vi "Full_Display.vi"() -> ()   [LabVIEW 2018]
uses:
  <vilib>/Utility/file.llb/Read Delimited Spreadsheet (DBL).vi
  D:/LocalElwood/localElwood/Manuals/SLM/SDK_from_1.1.0.84M/Blink_C_wrapper.dll
panel:
  out "Was it modified?":bool
  in  "stop 3":bool
  in  "stop 2":bool
  out "ok for com 2":bool
  out "new picture":picture
  in  "stop":bool
  in  "exit":bool
  in  "disconnect":bool
  in  "Divergence Button":bool
  in  "Orientation :":enum16{"Auto Orient", "0 Degrees", "45 Degress"}(ring)
  in  "1ovre on":bool
  in  "FWHM On":bool
  in  "Log on":bool
  in  "Gauss on":bool
  in  "1ovre":bool
  in  "FWHM":bool
  in  "Log":bool
  in  "Gauss":bool caption="Press to Activate Measurements"
  in  "Center :":enum16{"Centroid", "Peak"}(ring)
  in  "Display":T1(ring)=enum."3D Display" caption="Press Buttons to Activate XY Measurements"
  in  "Definition :":T2(ring)
  in  "Manual":bool
  in  "subtract background":bool caption="Capture"
  in  "Gray Scale":bool
  in  "mm":dbl=200.0 min=0.0 max=9999999.0
  in  "ms":dbl=50.0 min=0.06 max=200.0 step=0.01
  in  "Auto":bool=TRUE
  in  "Format Image":string(combo)="TXT"
  in  "save current image":bool caption="Capture"
  in  "start capture":bool caption="Capture"
  in  "connect":bool
  out "ok for com":bool
  out "Connected":bool
  out "Camera Serial Number":string
  out "PC Beamage Version":string caption="PC Beamage SW Version"
  out "Y Divergence":string
  out "X Divergence":string
  in  "Y Axis Measurements":T3(ring)=enum."Centroid"
  out "Y Axis Measurement":string caption="Y Axis Centroid"
  out "X Axis Measurement":string caption="X Axis Centroid"
  in  "X Axis Measurements":T3(ring)=enum."Centroid"
  in  "Common Measurements":T4(ring)=enum."Measure Effective Diameter"
  out "Common Measurement":string caption="Effective Diameter"
  in  "Time out":i32=-1
  out "DLL Present":bool=TRUE
  in  "Grating constant D\n    (0.2 by default)":dbl=0.2
  in  "Load angle_intensity":bool
  in  "Save angle_intensity":bool
  in  "main stop":bool
  in  "amp_angles":dbl=0.2
  in  "Order of pitch fork":dbl=1.0
  out "Pattern":picture
  out "File_title":string
  in  "Root Path":path=path "C:/localElwood/LabView/Magnet C006/Display_SLM_with_Zernike_Trigger_Beamprofiler_Bin"
  in  "LUT file location":string="C:\\Program Files\\Meadowlark Optics\\Blink 1920 HDMI\\LUT Files\\linear.blt"
  out "Status":dbl
  out "angle_intensity":dbl[](array[numeric])
  # "1\n2\n3\n4\n5\n6\n7\n8\n9\n10\n11\n12\n13\n14\n15\n16\n17\n18\n19\n20\n21\n22\n23\n24\n25\n26\n27\n28\n29\n30\n31\n32\n33\n34\n35\n36"
  # "* Remember to initialize angle_intensity, 0-1\n* Check the laser power is okay with 200ms fixed exposure time.\n* Check the root path is correct for this computer.\n* Check Z_num is initialized correctly."
  # "0"
  # "1"
  # "2"
  # "3"
  # "4"
  # "5"
  # "6"
  # "7"
  # "8"
  # "9"
  # "10"
  # "11"
  # "12"
  # "13"
  # "14"
  # "amp_angles defines the maximum\nintensity modulation you want to \napply. By default, it's 0.2."
  # "15"
  # "16"
  # "17"
  # "18"
  # "19"
  # "20"
  # "21"
  # "22"
  # "23"
  # "24"
  # "25"
  # "26"
  # "27"
  # "28"
  # "29"
  # "30"
  # "31"
  # "32"
  # "33"
  # "34"
  # "35"
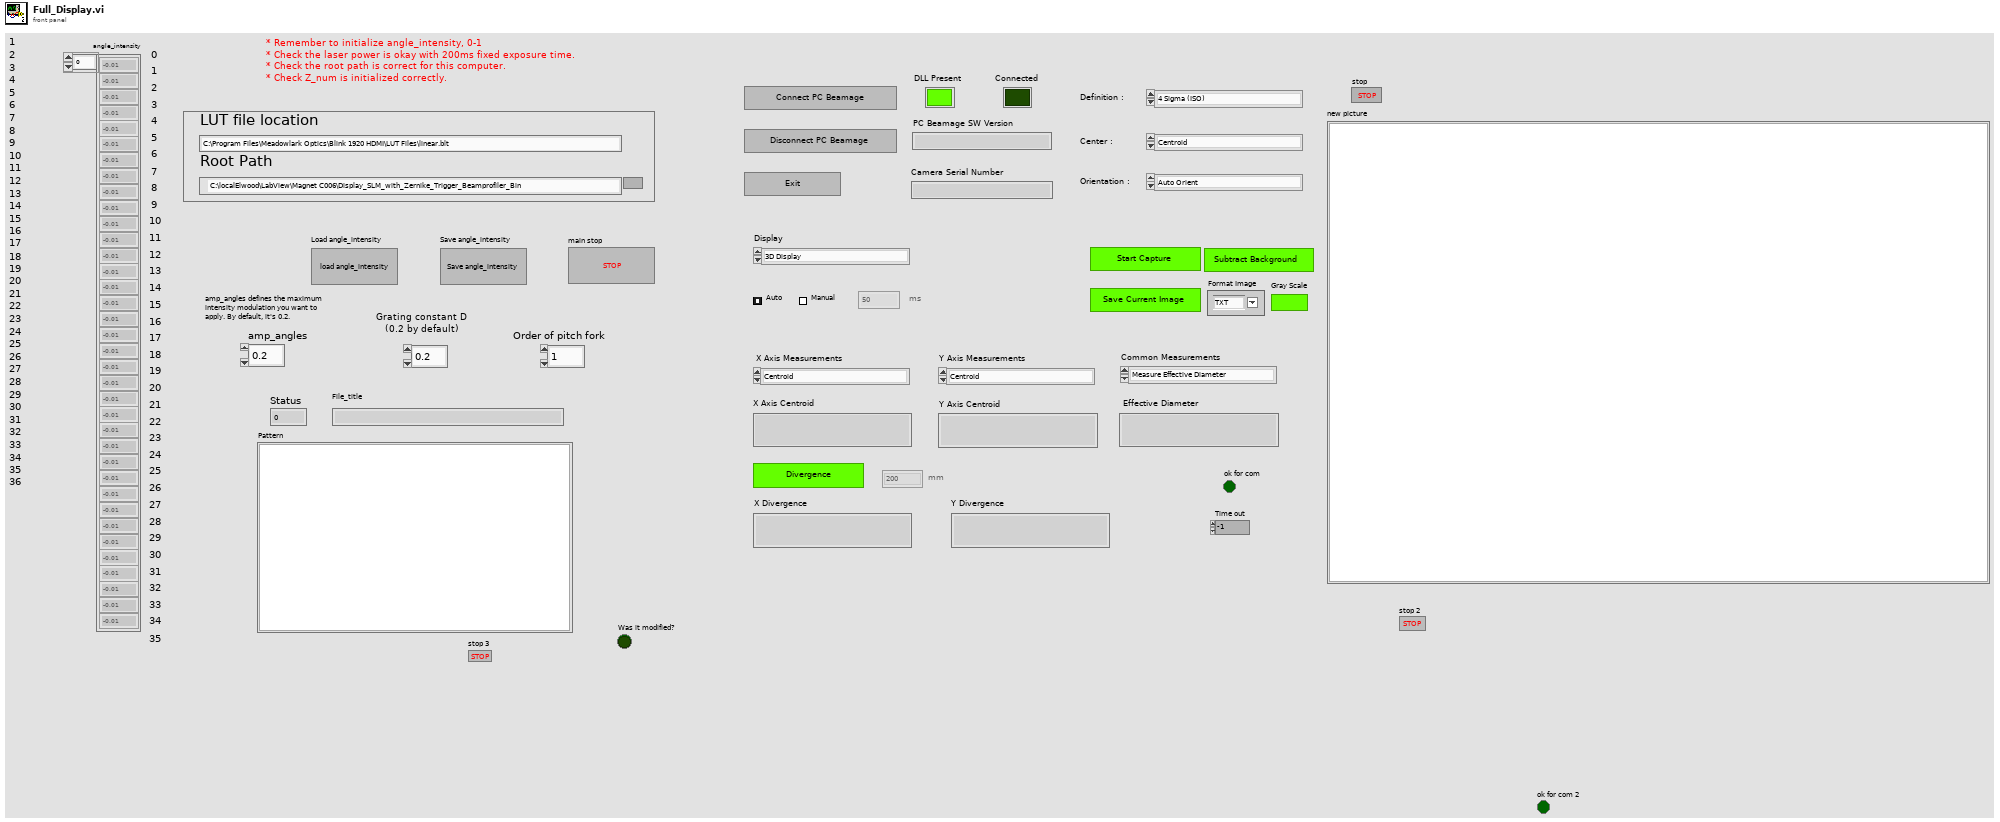
[diagram p1: front panel]
types:
  T1 = enum16{"2D Display", "3D Display", "XY Display", "Beam Track Display"}
  T2 = enum16{"4 Sigma (ISO)", "FWHM along Crosshairs (50%)", "1 / e^2 along Crosshairs (13.5%)", "86 % effective Diameter"}
  T3 = enum16{"1/e^2", "Centroid", "Delta", "FWHM", "Gaussian Equation", "Gaussian % Fit", "Roughness Fit", "Last", "Mean", "Peak to Average Ratio", "Peak"}
  T4 = enum16{"Measure Azimuth", "Measure Delta", "Measure Effective Diameter", "Measure Ellipticity", "Measure Number of Samples", "Measure Orientation", "Measure Peak Saturation", "Measure Minor Axis", "Measure Major Axis", "Measure RMS", ""}
  T5 = enum16{"open", "replace", "create", "open or create", "replace or create", "replace or create with confirmation"}
  T6 = typedef "LVBoundsTypeDef.ctl" = cluster{"Width":u32, "Height":u32}
  T7 = typedef "imagedata.ctl" = cluster{"image type":i32, "image depth":i32, "image":u8[], "mask":u8[], "colors":u32[], "Rectangle":cluster{"left":i16, "top":i16, "right":i16, "bottom":i16}}
  T8 = enum8{"Enabled", "Disabled", "Disabled and Grayed Out"}
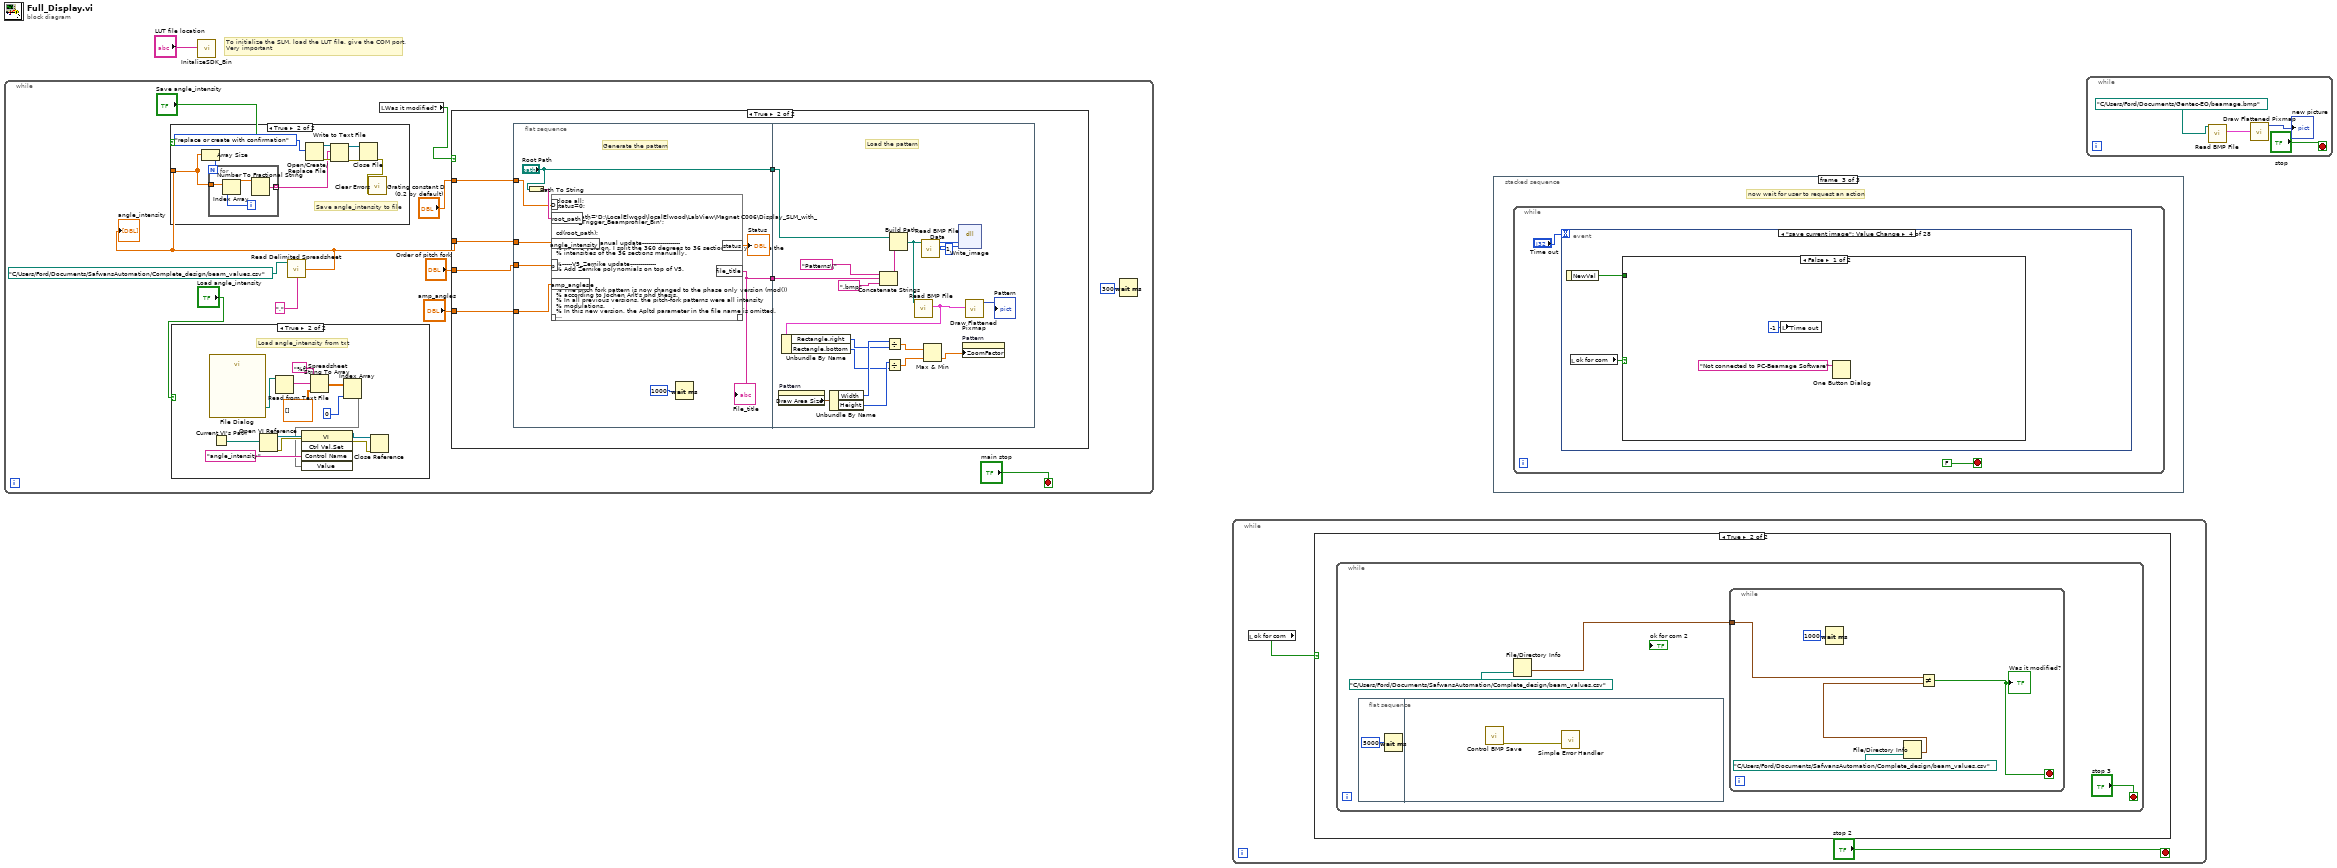
[diagram p0: block diagram]
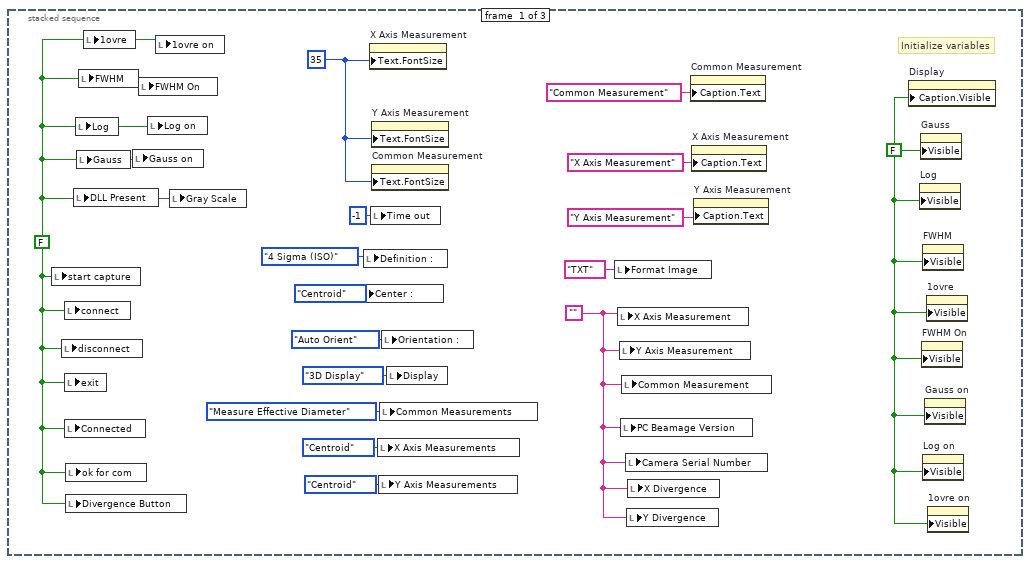
[diagram p3: hidden frame]
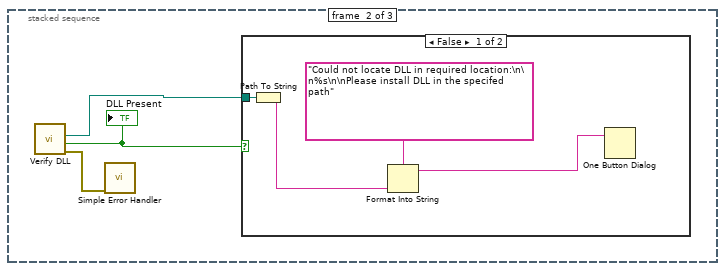
[diagram p4: hidden frame]
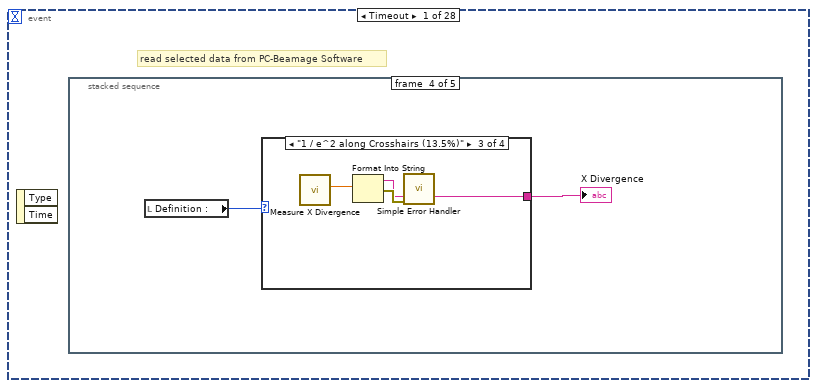
[diagram p6: hidden frame]
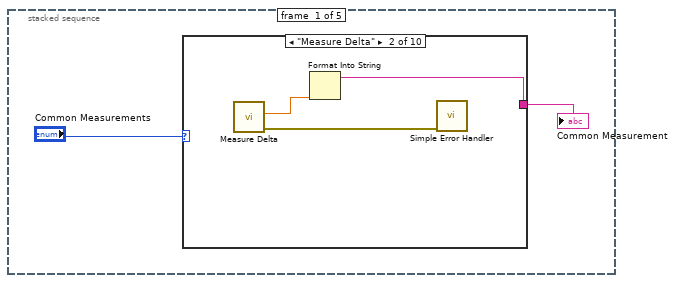
[diagram p7: hidden frame]
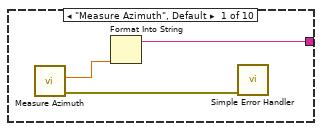
[diagram p8: hidden frame]
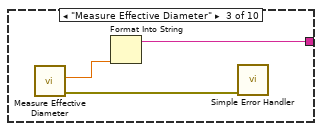
[diagram p9: hidden frame]
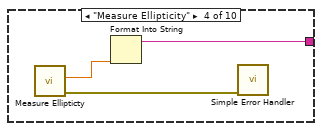
[diagram p10: hidden frame]
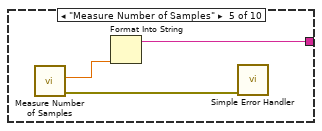
[diagram p11: hidden frame]
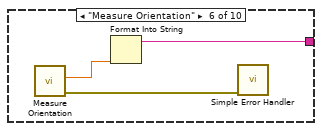
[diagram p12: hidden frame]
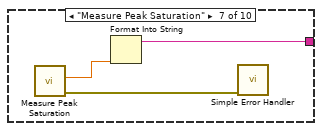
[diagram p13: hidden frame]
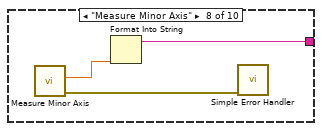
[diagram p14: hidden frame]
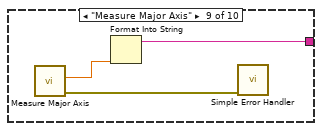
[diagram p15: hidden frame]
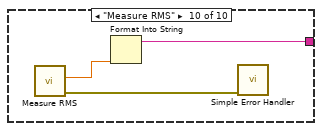
[diagram p16: hidden frame]
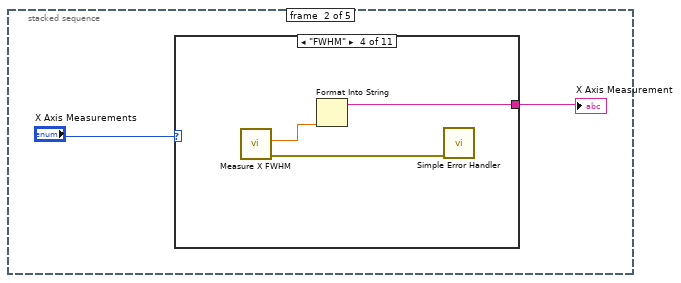
[diagram p17: hidden frame]
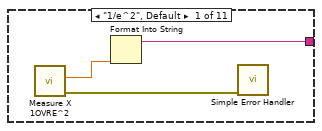
[diagram p18: hidden frame]
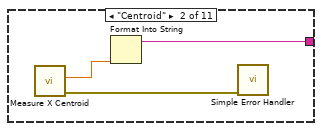
[diagram p19: hidden frame]
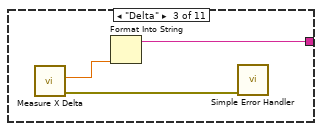
[diagram p20: hidden frame]
diagram:
  # "To initialize the SLM, load the LUT file, give the COM port.\nVery important"
  n1 = while {
    stop <- "main stop" stop-if-true
    n2 = case shown="True" "Load angle_intensity" {
      frame False {
      }
      frame True {
        # "Load angle_intensity from txt"
        n3 = call "File Dialog"() -> ("selected path"=w22:path)  [unwired: 12 in, 3 out]
        n4 = Current VI's Path() -> (path=w25:path)
        n5 = Open VI Reference(vi path=w25) -> (vi reference=w24:refnum<vi>, error out=w16:errorcluster)  [unwired: 5 in]
        n6 = Read from Text File(file (use dialog)=w22) -> (text=w21:string)  [unwired: 3 in, 3 out]
        n7 = Spreadsheet String To Array(format string="%f", spreadsheet string=w21, array type (2D Dbl)=dbl[][] []) -> (array=w13:dbl[][])  [unwired: 1 in]
        n8 = Index Array(array=w13, index (col)=0 ("disabled index (col)")) -> (element=w14:dbl[])  [unwired: 1 in]
        n9 = invoke class="VI" method="Ctrl Val.Set"(reference=w24, error in=w16, "Control Name"="angle_intensity", "Value"=w14) -> (reference out=w18:refnum<vi>, error out=w17:errorcluster)  [unwired: 1 in, 3 out]
        n10 = Close Reference(reference=w18, error in (no error)=w17) -> ()  [unwired: 1 out]
      }
    }
    n11 = call-poly <vilib>:"Read Delimited Spreadsheet.vi"("file path (dialog if empty)"=path "C:/Users/Ford/Documents/SafwansAutomation/Complete_design/beam_values.csv", "delimiter (\\t)"="," ("delimiter (\\t)")) -> ("first row"=w2:dbl[])  [unwired: 8 in, 5 out]
    "angle_intensity" <- w2
    n12 = case shown="True" "Save angle_intensity" {
      tunnel: w2 -> [_ w33]
      frame False {
      }
      frame True {
        # "Save angle_intensity to file"
        n13 = Array Size(array=w33) -> (size(s)=w34:i32)
        n14 = for {
          N: w34 -> [_]
          tunnel: w33 -> [w38]
          tunnel: [w35] -> w29 mode=indexing
          i -> [w37]
          n15 = Index Array(array=w38, index=w37) -> (element=w36:dbl)
          n16 = Number To Fractional String(number=w36) -> (F-format string=w35:string)  [unwired: 3 in]
        }
        n17 = Open/Create/Replace File(operation (0:open)=T5."replace or create with confirmation") -> (refnum out=w30:refnum<file>, error out=w31:errorcluster)  [unwired: 5 in, 1 out]
        n18 = Write to Text File(file (use dialog)=w30, text=w29, error in=w31) -> (refnum out=w27:refnum<file>, error out=w28:errorcluster)  [unwired: 1 in, 1 out]
        n19 = Close File(refnum=w27, error in=w28) -> (error out=w26:errorcluster)  [unwired: 1 out]
        n20 = call <vilib>:"Clear Errors.vi"("error in (no error)"=w26) -> ()  [unwired: 5 in, 2 out]
      }
    }
    n21 = local read "Was it modified?"() -> (w5:bool)
    n22 = case shown="True" w5 {
      tunnel: "amp_angles" -> [_ w42]
      tunnel: "Order of pitch fork" -> [_ w41]
      tunnel: w2 -> [_ w40]
      tunnel: "Grating constant D\n    (0.2 by default)" -> [_ w39]
      frame False {
      }
      frame True {
        n23 = flat-sequence {
          tunnel: w40 -> [w48]
          tunnel: [w51] -> w44
          tunnel: ["Root Path"] -> w43
          tunnel: w41 -> [w47]
          tunnel: w42 -> [w46]
          tunnel: w39 -> [w45]
          tunnel: w44 -> [w67]
          tunnel: w43 -> [w68]
          frame #0 {
            # "Generate the pattern"
            n24 = Path To String(path="Root Path") -> (string=w49:string)
            n25 = script code="close all;\nstatus=0;\n\n%root_path='D:\\LocalElwood\\localElwood\\LabView\\Magnet C006\\Display_SLM_with_Zernike_Trigger_Beamprofiler_Bin';\n\ncd(root_path);\n\n%--------------- manual update-------------------\n% In thie version, I split the 360 degrees to 36 sections and you tune the\n% intensities of the 36 sections manually.\n\n%-----V5_Zernike update-------------\n% Add Zernike polynomials on top of V5.\n\n\n%V5 update\n% The pitch fork pattern is now changed to the phase only version (mod())\n% according to Jochen Arlt's phd thesis.\n% In all previous versions, the pitch-fork patterns were all intensity\n% modulations.\n% In this new version, the Apltd parameter in the file name is omitted.\n\n\n%V4 update 2.\n% In order to average out the nonuniformity of the OAM beams intensity. V4\n% generates the pattern with a darkened region. In the SLM, the dsiplay\n% scans through all the pattersn and the averaged result should be uniform.\n\n%V4 update\n%The singularity of the pitch fork is now shifted to the position where\n%abbreation should be minumum. The position is found from the wavefront\n%correction bmp file.\n\n\n% V3 update, add amplitude and base, to maximize the 1st order diffraction\n% efficiency. Make the center hole area symmetric.\n% V2 update, change to the correct file format\n\n%Change two things\n% 1. p number\n% 2. r is the ratio between x and y axis. If r is not right, the center\n% hole for OAM light is not round. In other words, r is how much you strech\n% the piture.\n%Each time you want to generate a new picture, close the figure first!\n\n% The SLM only accept 8-bit grayscale pictures. 8-bit RGB does not work\n% with the SLM properly. Use colormap gray(256) to have the 8-bit grayscale\n% pictures.\n%% Basic paramters\n%D=0.2;\n%p=1;\nr=1.65;\nstrip_width=10;\namplitude=127.5; %127.5 correpsonds to the full range of SLM color 0-255. This helps to maximize the 1st order diffraction efficiency\nbase=0; %Defines where the base color is.\n\n%Z_num=[0,0,0,0,0,0,0,0,0,0,0,0,0,0];%No Z00, Z00 is always 1 in later code. [Z11,Z1-1,Z22,Z20,Z2-2,Z33,Z31,Z3-1,Z3-3,...Z4-4] from right to left on the wiki picture of Zernike polynomials\n%{\nangle_intensity=zeros(1,36);\namp_angles=0.2;\np=1;\n%}\n\n\nif size(angle_intensity)~=[1,36]\n    error('angle_intensity size wrong, should be [1,36]')\nend\n\n%%\nx=-10:(20/1919):10;  \ny=-(10/r):(20/r/1151):(10/r);\n\n[X,Y]=meshgrid(x,y);\n[theta,rho]=cart2pol(X,Y);\n\n\n%% Generate Zernike polynomials\n%The array size for the SLM is 17.6X10.7mm. Here we modulate the area of\n%diamter of 5mm\ndim=size(theta);\nr_max=4.5/17.6*10; %The radius of the area to cover. 4 should be the whole area of the beam. 4.5 is a safe number. Check \"Check_beam_diamter\" folder for more details.\n\n%% find the correponding index of the matrix for r_max. Will use them to reduce the amount of inversesinc calculation\nNN=zeros(1,2);MM=zeros(1,2);\nfor nn=2:dim(1)\n     if abs(y(nn-1))>=r_max&abs(y(nn))<r_max\n         NN(1,1)=nn-1;\n     elseif abs(y(nn-1))<=r_max&abs(y(nn))>r_max\n             NN(1,2)=nn+1;\n     end\nend\n\nfor mm=2:dim(2)\n     if abs(x(mm-1))>=r_max&abs(x(mm))<r_max\n         MM(1,1)=mm-1;\n     elseif abs(x(mm-1))<=r_max&abs(x(mm))>r_max\n             MM(1,2)=mm+1;\n     end\nend\n\n\n%%\nA_angles=zeros(dim(1),dim(2));\n\n\nxp=X(NN(1,1):NN(1,2),MM(1,1):MM(1,2));\nyp=Y(NN(1,1):NN(1,2),MM(1,1):MM(1,2));\n[theta_p,rho_p]=cart2pol(xp,yp);\nxp=xp.*heaviside(r_max-rho_p);\nyp=yp.*heaviside(r_max-rho_p);\ndim_p=size(theta_p);\n\nangle_intensity=[angle_intensity,angle_intensity(1,1)];% The value at angle=36 should be equal to angle=0\n\nposition=18+round(theta_p/(2*pi/36));\ntheta_p_amp=angle_intensity(1,position+1);\nA_angles(NN(1,1):NN(1,2),MM(1,1):MM(1,2))=reshape(theta_p_amp,[dim_p(1),dim_p(2)]);\n\n\n%{\nfigure (1)\nA_Zernike=A_Zernike.*heaviside(r_max-rho);\nsurf(X,Y,A_Zernike)\ngrid off\nshading flat\n%}\n\n\n%% Define the ideal amplitdue of the output beam you want\nA=(1-amp_angles)*ones(dim);\nA=(A+A_angles).*heaviside(r_max-rho);%Add a filter only the area inside the r_max regime is used.\nA=0.9*A./max(max(A)); % Normalized. This step will not make OAM+1 and -1 have the same power. You have the normilize the OAM+1 and -1 power in the last step.\n% The constant 0.9 is because the diffraction power is monotonic from 0-0.9.\n% Refer to \"Contolability_of_the_1st_order_power\" folder.\nB=inversesinc(A);\nM=1+1/pi.*B;\nF=2*pi/D*rho.*cos(theta)+p*theta-pi.*M;\nF=F.*heaviside(r_max-rho);%Add a filter only the area inside the r_max regime is used.\n\n\n%%------------Plot and save-----------\n%{\n    figure(2)\n\n    %surf(rho.*cos(theta),rho.*sin(theta),127.5*cos(2*pi/D*rho.*cos(theta)-p*theta)+127.5)\n    imagesc([-10 10],[-10,10],1/(2*pi)*M.*mod(F,2*pi)) %angle_step(theta,ratio).*\n    colormap(gray(256))\n    xlim([-10,10]);\n    ylim([-10,10])\n    grid off\n    shading interp\n    view(0,90)\n\n\n    set(gca,'XTickLabel',[]);\n    set(gca,'YTickLabel',[]);\n    set(gca,'xtick',[]);\n    set(gca,'ytick',[])\n%}\n\n    if p>0\n        file_title=['V5_p',num2str(abs(p)),'_D',num2str(D),'_8bit_r',num2str(r),'_Variable_angles'];\n    else\n        file_title=['V5_p',num2str(abs(p)),'_D',num2str(D),'_8bit_r',num2str(r),'_Variable_angles','_flipped'];\n    end\n\n    imwrite(2*amplitude*1/(2*pi)*M.*mod(F,2*pi),colormap(gray(256)),[root_path,'\\Patterns\\',file_title,'.bmp']);\n    status=1;\n\n    %It is quite important to use imwrite instead of print here. Imwrite\n    %offers the color scale option. Use gray(256), others do not work with the\n    %SLM.\n    %The factor 127.5 and the offset 127.5 is here to make the range 0-255 in\n    %order to match with the gray(256) color scale.\n    \n    %pause(1)\n    %close(1)"("root_path"=w49, "angle_intensity"=w48, "p"=w47, "amp_angles"=w46, "D"=w45) -> ("status"=→"Status":dbl, "file_title"=w51:string)  [unwired: 1 in, 1 out]
            "File_title" <- w51
            n26 = Wait (ms)(milliseconds to wait=u32 1000) -> ()  [unwired: 1 out]
          }
          frame #1 {
            # "Load the pattern"
            n27 = property on="Pattern" class="Pict"() -> ("Draw Area Size"=w61:T6)  [unwired: 2 in, 2 out]
            n28 = Unbundle By Name(w61) -> ("Width"=w60:u32, "Height"=w58:u32)
            n29 = Concatenate Strings("Patterns\\" ("string"), w67, ".bmp" ("name or relative path")) -> (w69:string)
            n30 = Build Path(base path=w68, name or relative path=w69) -> (appended path=w63:path)
            n31 = call <vilib>:"Read BMP File.vi"("path to BMP file"=w63) -> ("image data"=w62:T7)  [unwired: 8 in, 2 out]
            n32 = Unbundle By Name(w62) -> ("Rectangle.right"=w59:i16, "Rectangle.bottom"=w57:i16)
            n33 = Divide(x=w60, y=w59) -> (x/y=w56:dbl)
            n34 = Divide(x=w58, y=w57) -> (x/y=w55:dbl)
            n35 = call <vilib>:"Read BMP File Data.vi"("path to BMP file"=w63) -> ("BMP data"=w70:u8[])  [unwired: 6 in, 4 out]
            n36 = Max & Min(x=w56, y=w55) -> (min(x,y)=w54:dbl)  [unwired: 1 out]
            n37 = dll-call lib="D:/LocalElwood/localElwood/Manuals/SLM/SDK_from_1.1.0.84M/Blink_C_wrapper.dll" fn="Write_image"("image_data"=w70, "isEightBit"=i8 1) -> ()  [unwired: 6 in, 2 out]
            n38 = property on="Pattern" class="Pict"("ZoomFactor"=w54) -> ()  [unwired: 2 in, 2 out]
            n39 = call <vilib>:"Draw Flattened Pixmap.vi"("image data"=w62) -> ("new picture"=→"Pattern":picture)  [unwired: 8 in]
          }
        }
      }
    }
    n40 = Wait (ms)(milliseconds to wait=u32 300) -> ()  [unwired: 1 out]
  }
  n41 = call "InitalizeSDK_Bin.vi"("LUT file location"="LUT file location") -> ()
  n42 = while {
    stop <- "stop 2" stop-if-true
    n43 = local read "ok for com"() -> (w73:bool)
    n44 = case shown="True" w73 {
      frame False {
      }
      frame True {
        n45 = while {
          stop <- "stop 3" stop-if-true
          n46 = flat-sequence {
            frame #0 {
              n47 = Wait (ms)(milliseconds to wait=u32 5000) -> ()  [unwired: 1 out]
            }
            frame #1 {
              n48 = call "Control BMP Save.vi"() -> ("error out"=w78:errorcluster)  [unwired: 9 in, 2 out]
              n49 = call <vilib>:"Simple Error Handler.vi"("error in (no error)"=w78) -> ()  [unwired: 4 in, 5 out]
            }
          }
          n50 = File/Directory Info(path=path "C:/Users/Ford/Documents/SafwansAutomation/Complete_design/beam_values.csv") -> (last mod=w75:timestamp)  [unwired: 1 in, 6 out]
          n51 = while {
            tunnel: w75 -> [w82]
            stop <- w80 stop-if-true
            n52 = Wait (ms)(milliseconds to wait=u32 1000) -> ()  [unwired: 1 out]
            n53 = File/Directory Info(path=path "C:/Users/Ford/Documents/SafwansAutomation/Complete_design/beam_values.csv") -> (last mod=w81:timestamp)  [unwired: 1 in, 6 out]
            n54 = Not Equal?(x=w82, y=w81) -> (x != y?=w80:bool)
            "Was it modified?" <- w80
          }
        }
      }
    }
  }
  n55 = stacked-sequence {
    frame #0 {
      w89 = FALSE ("Visible")
      w92 = u32 35 ("Text.Font:Size")
      w84 = FALSE ("verifiy dll")
      w86 = ""
      # "Initialize variables"
      n56 = local write "start capture"(w84) -> ()
      n57 = local write "disconnect"(w84) -> ()
      n58 = local write "connect"(w84) -> ()
      n59 = local write "exit"(w84) -> ()
      n60 = local write "Connected"(w84) -> ()
      n61 = local write "ok for com"(w84) -> ()
      n62 = local write "Divergence Button"(w84) -> ()
      n63 = local write "DLL Present"(w84) -> ()
      n64 = local write "Log"(w84) -> ()
      n65 = local write "Gauss"(w84) -> ()
      n66 = local write "FWHM"(w84) -> ()
      n67 = local write "1ovre"(w84) -> ()
      n68 = local write "Gauss on"(w84) -> ()
      n69 = local write "FWHM On"(w84) -> ()
      n70 = local write "Log on"(w84) -> ()
      n71 = local write "1ovre on"(w84) -> ()
      n72 = local write "Gray Scale"(w84) -> ()
      n73 = local write "Center :"(enum16{"Centroid", "Peak"}."Centroid" ("Center :")) -> ()
      n74 = local write "Definition :"(T2."4 Sigma (ISO)" ("Definition :")) -> ()
      n75 = property on="X Axis Measurement" class="Str"("Text.FontSize"=w92) -> ()  [unwired: 2 in, 2 out]
      n76 = local write "Time out"(-1 ("Time out")) -> ()
      n77 = property on="Y Axis Measurement" class="Str"("Text.FontSize"=w92) -> ()  [unwired: 2 in, 2 out]
      n78 = property on="Common Measurement" class="Str"("Text.FontSize"=w92) -> ()  [unwired: 2 in, 2 out]
      n79 = local write "X Axis Measurements"(T3."Centroid" ("X Axis Measurements")) -> ()
      n80 = local write "Y Axis Measurements"(T3."Centroid" ("Y Axis Measurements")) -> ()
      n81 = local write "Common Measurements"(T4."Measure Effective Diameter" ("Common Measurements")) -> ()
      n82 = local write "Orientation :"(enum16{"Auto Orient", "0 Degrees", "45 Degress"}."Auto Orient" ("Orientation :")) -> ()
      n83 = local write "Display"(T1."3D Display" ("Display")) -> ()
      n84 = local write "Format Image"("TXT" ("Format Image")) -> ()
      n85 = local write "X Axis Measurement"(w86) -> ()
      n86 = local write "Y Axis Measurement"(w86) -> ()
      n87 = local write "PC Beamage Version"(w86) -> ()
      n88 = local write "Common Measurement"(w86) -> ()
      n89 = local write "Camera Serial Number"(w86) -> ()
      n90 = local write "Y Divergence"(w86) -> ()
      n91 = local write "X Divergence"(w86) -> ()
      n92 = property on="Common Measurement" class="Str"("Caption.Text"="Common Measurement") -> ()  [unwired: 2 in, 2 out]
      n93 = property on="X Axis Measurement" class="Str"("Caption.Text"="X Axis Measurement") -> ()  [unwired: 2 in, 2 out]
      n94 = property on="Y Axis Measurement" class="Str"("Caption.Text"="Y Axis Measurement") -> ()  [unwired: 2 in, 2 out]
      n95 = property on="Display" class="Enum (strict)"("Caption.Visible"=w89) -> ()  [unwired: 2 in, 2 out]
      n96 = property on="Log" class="Bool (strict)"("Visible"=w89) -> ()  [unwired: 2 in, 2 out]
      n97 = property on="Gauss" class="Bool (strict)"("Visible"=w89) -> ()  [unwired: 2 in, 2 out]
      n98 = property on="FWHM On" class="Bool (strict)"("Visible"=w89) -> ()  [unwired: 2 in, 2 out]
      n99 = property on="FWHM" class="Bool (strict)"("Visible"=w89) -> ()  [unwired: 2 in, 2 out]
      n100 = property on="Log on" class="Bool (strict)"("Visible"=w89) -> ()  [unwired: 2 in, 2 out]
      n101 = property on="Gauss on" class="Bool (strict)"("Visible"=w89) -> ()  [unwired: 2 in, 2 out]
      n102 = property on="1ovre" class="Bool (strict)"("Visible"=w89) -> ()  [unwired: 2 in, 2 out]
      n103 = property on="1ovre on" class="Bool (strict)"("Visible"=w89) -> ()  [unwired: 2 in, 2 out]
    }
    frame #1 {
      n104 = call "Verify DLL.vi"() -> ("error out"=w100:errorcluster, "DLL is Present"=w102:bool, "path"=w101:path)  [unwired: 9 in]
      "DLL Present" <- w102
      n105 = call <vilib>:"Simple Error Handler.vi"("error in (no error)"=w100) -> ()  [unwired: 4 in, 5 out]
      n106 = case shown="False" w102 {
        tunnel: w101 -> [w106 _]
        frame False {
          n107 = Path To String(path=w106) -> (string=w104:string)
          n108 = Format Into String(format string="Could not locate DLL in required location:\n\n%s\n\nPlease install DLL in the specifed path", w104) -> (resulting string=w103:string)  [unwired: 2 in, 1 out]
          n109 = One Button Dialog(message=w103) -> ()  [unwired: 1 in, 1 out]
        }
        frame True {
        }
      }
    }
    frame #2 {
      # "now wait for user to request an action"
      n110 = while {
        stop <- FALSE stop-if-true
        n111 = event shown="[3] \"save current image\": Value Change" {
          selector: _ -> [_ _ _ _ _ _ _ _ _ _ _ _ _ _ _ _ _ _ _ _ _ _ _ _ _ _ _ _]
          dyn-events: _ -> [_ _ _ _ _ _ _ _ _ _ _ _ _ _ _ _ _ _ _ _ _ _ _ _ _ _ _ _]
          timeout: "Time out" -> [_ _ _ _ _ _ _ _ _ _ _ _ _ _ _ _ _ _ _ _ _ _ _ _ _ _ _ _]
          event Timeout {
            # "read selected data from PC-Beamage Software"
            n112 = event-data() -> ()  [unwired: 1 in, 2 out]
            n113 = stacked-sequence {
              frame #0 {
                n114 = case shown="\"Measure Delta\"" "Common Measurements" {
                  tunnel: [w111 w114 w117 w120 w123 w126 w129 w132 w135 w138] -> w109
                  frame "Measure Azimuth", Default {
                    n115 = call "Measure Azimuth.vi"() -> ("error out"=w113:errorcluster, "Azimuth"=w112:dbl)  [unwired: 10 in]
                    n116 = Format Into String(w112) -> (resulting string=w111:string)  [unwired: 3 in, 1 out]
                    n117 = call <vilib>:"Simple Error Handler.vi"("error in (no error)"=w113) -> ()  [unwired: 4 in, 5 out]
                  }
                  frame "Measure Delta" {
                    n118 = call "Measure Delta.vi"() -> ("error out"=w116:errorcluster, "Delta"=w115:dbl)  [unwired: 10 in]
                    n119 = Format Into String(w115) -> (resulting string=w114:string)  [unwired: 3 in, 1 out]
                    n120 = call <vilib>:"Simple Error Handler.vi"("error in (no error)"=w116) -> ()  [unwired: 4 in, 5 out]
                  }
                  frame "Measure Effective Diameter" {
                    n121 = call "Measure Effective Diameter.vi"() -> ("error out"=w119:errorcluster, "Effective Diameter"=w118:dbl)  [unwired: 10 in]
                    n122 = Format Into String(w118) -> (resulting string=w117:string)  [unwired: 3 in, 1 out]
                    n123 = call <vilib>:"Simple Error Handler.vi"("error in (no error)"=w119) -> ()  [unwired: 4 in, 5 out]
                  }
                  frame "Measure Ellipticity" {
                    n124 = call "Measure Ellipticty.vi"() -> ("error out"=w122:errorcluster, "Ellipticity"=w121:dbl)  [unwired: 10 in]
                    n125 = Format Into String(w121) -> (resulting string=w120:string)  [unwired: 3 in, 1 out]
                    n126 = call <vilib>:"Simple Error Handler.vi"("error in (no error)"=w122) -> ()  [unwired: 4 in, 5 out]
                  }
                  frame "Measure Number of Samples" {
                    n127 = call "Measure Number of Samples.vi"() -> ("error out"=w125:errorcluster, "Number of Samples"=w124:dbl)  [unwired: 10 in]
                    n128 = Format Into String(w124) -> (resulting string=w123:string)  [unwired: 3 in, 1 out]
                    n129 = call <vilib>:"Simple Error Handler.vi"("error in (no error)"=w125) -> ()  [unwired: 4 in, 5 out]
                  }
                  frame "Measure Orientation" {
                    n130 = call "Measure Orientation.vi"() -> ("error out"=w128:errorcluster, "Orienttion"=w127:dbl)  [unwired: 10 in]
                    n131 = Format Into String(w127) -> (resulting string=w126:string)  [unwired: 3 in, 1 out]
                    n132 = call <vilib>:"Simple Error Handler.vi"("error in (no error)"=w128) -> ()  [unwired: 4 in, 5 out]
                  }
                  frame "Measure Peak Saturation" {
                    n133 = call "Measure Peak Saturation.vi"() -> ("error out"=w131:errorcluster, "Peak Saturation"=w130:dbl)  [unwired: 10 in]
                    n134 = Format Into String(w130) -> (resulting string=w129:string)  [unwired: 3 in, 1 out]
                    n135 = call <vilib>:"Simple Error Handler.vi"("error in (no error)"=w131) -> ()  [unwired: 4 in, 5 out]
                  }
                  frame "Measure Minor Axis" {
                    n136 = call "Measure Minor Axis.vi"() -> ("error out"=w134:errorcluster, "Minor Axis"=w133:dbl)  [unwired: 10 in]
                    n137 = Format Into String(w133) -> (resulting string=w132:string)  [unwired: 3 in, 1 out]
                    n138 = call <vilib>:"Simple Error Handler.vi"("error in (no error)"=w134) -> ()  [unwired: 4 in, 5 out]
                  }
                  frame "Measure Major Axis" {
                    n139 = call "Measure Major Axis.vi"() -> ("error out"=w137:errorcluster, "Major Axis"=w136:dbl)  [unwired: 10 in]
                    n140 = Format Into String(w136) -> (resulting string=w135:string)  [unwired: 3 in, 1 out]
                    n141 = call <vilib>:"Simple Error Handler.vi"("error in (no error)"=w137) -> ()  [unwired: 4 in, 5 out]
                  }
                  frame "Measure RMS" {
                    n142 = call "Measure RMS.vi"() -> ("error out"=w140:errorcluster, "RMS"=w139:dbl)  [unwired: 10 in]
                    n143 = Format Into String(w139) -> (resulting string=w138:string)  [unwired: 3 in, 1 out]
                    n144 = call <vilib>:"Simple Error Handler.vi"("error in (no error)"=w140) -> ()  [unwired: 4 in, 5 out]
                  }
                }
                "Common Measurement" <- w109
              }
              frame #1 {
                n145 = case shown="\"FWHM\"" "X Axis Measurements" {
                  tunnel: [w143 w146 w149 w152 w155 w159 w162 w165 w168 w171 w174] -> w141
                  frame "1/e^2", Default {
                    n146 = call "Measure X 1OVRE^2.vi"() -> ("error out"=w145:errorcluster, "X 1/E^2"=w144:dbl)  [unwired: 10 in]
                    n147 = Format Into String(w144) -> (resulting string=w143:string)  [unwired: 3 in, 1 out]
                    n148 = call <vilib>:"Simple Error Handler.vi"("error in (no error)"=w145) -> ()  [unwired: 4 in, 5 out]
                  }
                  frame "Centroid" {
                    n149 = call "Measure X Centroid.vi"() -> ("error out"=w148:errorcluster, "X Centroid"=w147:dbl)  [unwired: 10 in]
                    n150 = Format Into String(w147) -> (resulting string=w146:string)  [unwired: 3 in, 1 out]
                    n151 = call <vilib>:"Simple Error Handler.vi"("error in (no error)"=w148) -> ()  [unwired: 4 in, 5 out]
                  }
                  frame "Delta" {
                    n152 = call "Measure X Delta.vi"() -> ("error out"=w151:errorcluster, "X Delta"=w150:dbl)  [unwired: 10 in]
                    n153 = Format Into String(w150) -> (resulting string=w149:string)  [unwired: 3 in, 1 out]
                    n154 = call <vilib>:"Simple Error Handler.vi"("error in (no error)"=w151) -> ()  [unwired: 4 in, 5 out]
                  }
                  frame "FWHM" {
                    n155 = call "Measure X FWHM.vi"() -> ("error out"=w154:errorcluster, "X FWHM"=w153:dbl)  [unwired: 10 in]
                    n156 = Format Into String(w153) -> (resulting string=w152:string)  [unwired: 3 in, 1 out]
                    n157 = call <vilib>:"Simple Error Handler.vi"("error in (no error)"=w154) -> ()  [unwired: 4 in, 5 out]
                  }
                  frame "Gaussian Equation" {
                    n158 = call "Measure X Gaussian Equation.vi"() -> ("error out"=w158:errorcluster, "X Gaussian Equation"=w157:string)  [unwired: 10 in]
                    n159 = Match Pattern(string=w157, regular expression=":") -> (after substring=w155:string)  [unwired: 1 in, 3 out]
                    n160 = call <vilib>:"Simple Error Handler.vi"("error in (no error)"=w158) -> ()  [unwired: 4 in, 5 out]
                  }
                  frame "Gaussian % Fit" {
                    n161 = call "Measure X Gaussian Fit %.vi"() -> ("error out"=w161:errorcluster, "X Gaussian Fit %"=w160:dbl)  [unwired: 10 in]
                    n162 = Format Into String(w160) -> (resulting string=w159:string)  [unwired: 3 in, 1 out]
                    n163 = call <vilib>:"Simple Error Handler.vi"("error in (no error)"=w161) -> ()  [unwired: 4 in, 5 out]
                  }
                  frame "Roughness Fit" {
                    n164 = call "Measure X Roughness Fit.vi"() -> ("error out"=w164:errorcluster, "X Roughness Fit"=w163:dbl)  [unwired: 10 in]
                    n165 = Format Into String(w163) -> (resulting string=w162:string)  [unwired: 3 in, 1 out]
                    n166 = call <vilib>:"Simple Error Handler.vi"("error in (no error)"=w164) -> ()  [unwired: 4 in, 5 out]
                  }
                  frame "Last" {
                    n167 = call "Measure X Last.vi"() -> ("error out"=w167:errorcluster, "X Last"=w166:dbl)  [unwired: 10 in]
                    n168 = Format Into String(w166) -> (resulting string=w165:string)  [unwired: 3 in, 1 out]
                    n169 = call <vilib>:"Simple Error Handler.vi"("error in (no error)"=w167) -> ()  [unwired: 4 in, 5 out]
                  }
                  frame "Mean" {
                    n170 = call "Measure Y Divergence.vi"() -> ("error out"=w170:errorcluster, "X Mean"=w169:dbl)  [unwired: 10 in]
                    n171 = Format Into String(w169) -> (resulting string=w168:string)  [unwired: 3 in, 1 out]
                    n172 = call <vilib>:"Simple Error Handler.vi"("error in (no error)"=w170) -> ()  [unwired: 4 in, 5 out]
                  }
                  frame "Peak to Average Ratio" {
                    n173 = call "Measure X Peak to Average.vi"() -> ("error out"=w173:errorcluster, "X Peak to Average Ratio"=w172:dbl)  [unwired: 10 in]
                    n174 = Format Into String(w172) -> (resulting string=w171:string)  [unwired: 3 in, 1 out]
                    n175 = call <vilib>:"Simple Error Handler.vi"("error in (no error)"=w173) -> ()  [unwired: 4 in, 5 out]
                  }
                  frame "Peak" {
                    n176 = call "Measure X Peak.vi"() -> ("error out"=w176:errorcluster, "X Peak"=w175:dbl)  [unwired: 10 in]
                    n177 = Format Into String(w175) -> (resulting string=w174:string)  [unwired: 3 in, 1 out]
                    n178 = call <vilib>:"Simple Error Handler.vi"("error in (no error)"=w176) -> ()  [unwired: 4 in, 5 out]
                  }
                }
                "X Axis Measurement" <- w141
              }
              frame #2 {
                n179 = case shown="\"Gaussian Equation\"" "Y Axis Measurements" {
                  tunnel: [w179 w182 w185 w188 w191 w195 w198 w201 w204 w207 w210] -> w177
                  frame "1/e^2", Default {
                    n180 = call "Measure Y 1OVRE^2.vi"() -> ("error out"=w181:errorcluster, "Y 1/E^2"=w180:dbl)  [unwired: 10 in]
                    n181 = Format Into String(w180) -> (resulting string=w179:string)  [unwired: 3 in, 1 out]
                    n182 = call <vilib>:"Simple Error Handler.vi"("error in (no error)"=w181) -> ()  [unwired: 4 in, 5 out]
                  }
                  frame "Centroid" {
                    n183 = call "Measure Y Centroid.vi"() -> ("error out"=w184:errorcluster, "Y Centroid"=w183:dbl)  [unwired: 10 in]
                    n184 = Format Into String(w183) -> (resulting string=w182:string)  [unwired: 3 in, 1 out]
                    n185 = call <vilib>:"Simple Error Handler.vi"("error in (no error)"=w184) -> ()  [unwired: 4 in, 5 out]
                  }
                  frame "Delta" {
                    n186 = call "Measure Y Delta.vi"() -> ("error out"=w187:errorcluster, "Y Delta"=w186:dbl)  [unwired: 10 in]
                    n187 = Format Into String(w186) -> (resulting string=w185:string)  [unwired: 3 in, 1 out]
                    n188 = call <vilib>:"Simple Error Handler.vi"("error in (no error)"=w187) -> ()  [unwired: 4 in, 5 out]
                  }
                  frame "FWHM" {
                    n189 = call "Measure Y FWHM.vi"() -> ("error out"=w190:errorcluster, "Y FWHM"=w189:dbl)  [unwired: 10 in]
                    n190 = Format Into String(w189) -> (resulting string=w188:string)  [unwired: 3 in, 1 out]
                    n191 = call <vilib>:"Simple Error Handler.vi"("error in (no error)"=w190) -> ()  [unwired: 4 in, 5 out]
                  }
                  frame "Gaussian Equation" {
                    n192 = call "Measure Y Gaussian Equation.vi"() -> ("error out"=w194:errorcluster, "Y Gaussian Equation"=w193:string)  [unwired: 10 in]
                    n193 = Match Pattern(string=w193, regular expression=": ") -> (after substring=w191:string)  [unwired: 1 in, 3 out]
                    n194 = call <vilib>:"Simple Error Handler.vi"("error in (no error)"=w194) -> ()  [unwired: 4 in, 5 out]
                  }
                  frame "Gaussian % Fit" {
                    n195 = call "Measure Y Gaussian Fit %.vi"() -> ("error out"=w197:errorcluster, "Y Gaussian Fit %"=w196:dbl)  [unwired: 10 in]
                    n196 = Format Into String(w196) -> (resulting string=w195:string)  [unwired: 3 in, 1 out]
                    n197 = call <vilib>:"Simple Error Handler.vi"("error in (no error)"=w197) -> ()  [unwired: 4 in, 5 out]
                  }
                  frame "Roughness Fit" {
                    n198 = call "Measure Y Roughness Fit.vi"() -> ("error out"=w200:errorcluster, "Y Roughness Fit"=w199:dbl)  [unwired: 10 in]
                    n199 = Format Into String(w199) -> (resulting string=w198:string)  [unwired: 3 in, 1 out]
                    n200 = call <vilib>:"Simple Error Handler.vi"("error in (no error)"=w200) -> ()  [unwired: 4 in, 5 out]
                  }
                  frame "Last" {
                    n201 = call "Measure Y Last.vi"() -> ("error out"=w203:errorcluster, "Y Last"=w202:dbl)  [unwired: 10 in]
                    n202 = Format Into String(w202) -> (resulting string=w201:string)  [unwired: 3 in, 1 out]
                    n203 = call <vilib>:"Simple Error Handler.vi"("error in (no error)"=w203) -> ()  [unwired: 4 in, 5 out]
                  }
                  frame "Mean" {
                    n204 = call "Measure Y Mean.vi"() -> ("error out"=w206:errorcluster, "Y Mean"=w205:dbl)  [unwired: 10 in]
                    n205 = Format Into String(w205) -> (resulting string=w204:string)  [unwired: 3 in, 1 out]
                    n206 = call <vilib>:"Simple Error Handler.vi"("error in (no error)"=w206) -> ()  [unwired: 4 in, 5 out]
                  }
                  frame "Peak to Average Ratio" {
                    n207 = call "Measure Y Peak to Average.vi"() -> ("error out"=w209:errorcluster, "Y Peak to Average Ratio"=w208:dbl)  [unwired: 10 in]
                    n208 = Format Into String(w208) -> (resulting string=w207:string)  [unwired: 3 in, 1 out]
                    n209 = call <vilib>:"Simple Error Handler.vi"("error in (no error)"=w209) -> ()  [unwired: 4 in, 5 out]
                  }
                  frame "Peak" {
                    n210 = call "Measure Y Peak.vi"() -> ("error out"=w212:errorcluster, "Y Peak"=w211:dbl)  [unwired: 10 in]
                    n211 = Format Into String(w211) -> (resulting string=w210:string)  [unwired: 3 in, 1 out]
                    n212 = call <vilib>:"Simple Error Handler.vi"("error in (no error)"=w212) -> ()  [unwired: 4 in, 5 out]
                  }
                }
                "Y Axis Measurement" <- w177
              }
              frame #3 {
                n213 = local read "Definition :"() -> (w214:T2)
                n214 = case shown="\"1 / e^2 along Crosshairs (13.5%)\"" w214 {
                  tunnel: [w215 w218 w221 w224] -> w213
                  frame "4 Sigma (ISO)", Default {
                    n215 = call "Measure X Divergence.vi"() -> ("X Mean"=w217:dbl)  [unwired: 10 in, 1 out]
                    n216 = Format Into String(w217) -> (resulting string=w215:string, error out=w216:errorcluster)  [unwired: 3 in]
                    n217 = call <vilib>:"Simple Error Handler.vi"("error in (no error)"=w216) -> ()  [unwired: 4 in, 5 out]
                  }
                  frame "FWHM along Crosshairs (50%)" {
                    n218 = call "Measure X Divergence.vi"() -> ("X Mean"=w220:dbl)  [unwired: 10 in, 1 out]
                    n219 = Format Into String(w220) -> (resulting string=w218:string, error out=w219:errorcluster)  [unwired: 3 in]
                    n220 = call <vilib>:"Simple Error Handler.vi"("error in (no error)"=w219) -> ()  [unwired: 4 in, 5 out]
                  }
                  frame "1 / e^2 along Crosshairs (13.5%)" {
                    n221 = call "Measure X Divergence.vi"() -> ("X Mean"=w223:dbl)  [unwired: 10 in, 1 out]
                    n222 = Format Into String(w223) -> (resulting string=w221:string, error out=w222:errorcluster)  [unwired: 3 in]
                    n223 = call <vilib>:"Simple Error Handler.vi"("error in (no error)"=w222) -> ()  [unwired: 4 in, 5 out]
                  }
                  frame "86 % effective Diameter" {
                    n224 = call "Measure X Divergence.vi"() -> ("X Mean"=w226:dbl)  [unwired: 10 in, 1 out]
                    n225 = Format Into String(w226) -> (resulting string=w224:string, error out=w225:errorcluster)  [unwired: 3 in]
                    n226 = call <vilib>:"Simple Error Handler.vi"("error in (no error)"=w225) -> ()  [unwired: 4 in, 5 out]
                  }
                }
                "X Divergence" <- w213
              }
              frame #4 {
                n227 = local read "Definition :"() -> (w228:T2)
                n228 = case shown="\"4 Sigma (ISO)\", Default" w228 {
                  tunnel: [w229 w232 w235 w238] -> w227
                  frame "4 Sigma (ISO)", Default {
                    n229 = call "Measure Y Divergence.vi"() -> ("X Mean"=w231:dbl)  [unwired: 10 in, 1 out]
                    n230 = Format Into String(w231) -> (resulting string=w229:string, error out=w230:errorcluster)  [unwired: 3 in]
                    n231 = call <vilib>:"Simple Error Handler.vi"("error in (no error)"=w230) -> ()  [unwired: 4 in, 5 out]
                  }
                  frame "FWHM along Crosshairs (50%)" {
                    n232 = call "Measure Y Divergence.vi"() -> ("X Mean"=w234:dbl)  [unwired: 10 in, 1 out]
                    n233 = Format Into String(w234) -> (resulting string=w232:string, error out=w233:errorcluster)  [unwired: 3 in]
                    n234 = call <vilib>:"Simple Error Handler.vi"("error in (no error)"=w233) -> ()  [unwired: 4 in, 5 out]
                  }
                  frame "1 / e^2 along Crosshairs (13.5%)" {
                    n235 = call "Measure Y Divergence.vi"() -> ("X Mean"=w237:dbl)  [unwired: 10 in, 1 out]
                    n236 = Format Into String(w237) -> (resulting string=w235:string, error out=w236:errorcluster)  [unwired: 3 in]
                    n237 = call <vilib>:"Simple Error Handler.vi"("error in (no error)"=w236) -> ()  [unwired: 4 in, 5 out]
                  }
                  frame "86 % effective Diameter" {
                    n238 = call "Measure Y Divergence.vi"() -> ("X Mean"=w240:dbl)  [unwired: 10 in, 1 out]
                    n239 = Format Into String(w240) -> (resulting string=w238:string, error out=w239:errorcluster)  [unwired: 3 in]
                    n240 = call <vilib>:"Simple Error Handler.vi"("error in (no error)"=w239) -> ()  [unwired: 4 in, 5 out]
                  }
                }
                "Y Divergence" <- w227
              }
            }
          }
          event "connect": Value Change {
            n241 = event-data() -> ()  [unwired: 1 in, 1 out]
            n242 = stacked-sequence {
              frame #0 {
                n243 = call "Connect to PC Beamage 64 bit DLL.vi"() -> ("error out"=w242:errorcluster, "Connected"=w243:bool)  [unwired: 10 in]
                "Connected" <- w243
                n244 = case shown="True" w243 {
                  tunnel: w242 -> [w245 w247]
                  tunnel: [w245 w250] -> w241
                  frame False {
                    n245 = One Button Dialog(message="Connection Failed. Verify PC Beamage 3.0 is\nrunning and the Labview Pipe is Open.\n\nShow/Hide\n  Options\n>Start Labview Pipeline") -> ()  [unwired: 1 in, 1 out]
                  }
                  frame True {
                    n246 = call "Control Stop Capture.vi"("error in"=w247) -> ("error out"=w246:errorcluster)  [unwired: 8 in, 2 out]
                    n247 = call "Query PC Beamage Version.vi"("error in"=w246) -> ("error out"=w251:errorcluster, "PC Beamage Version"=→"PC Beamage Version":string)  [unwired: 9 in]
                    n248 = call "Query Serial Number.vi"("error in"=w251) -> ("error out"=w250:errorcluster, "Serial Number"=→"Camera Serial Number":string)  [unwired: 9 in]
                  }
                }
                n249 = call <vilib>:"Simple Error Handler.vi"("error in (no error)"=w241) -> ()  [unwired: 4 in, 5 out]
              }
              frame #1 {
                w252 = FALSE ("verifiy dll")
                n250 = local read "Connected"() -> (w254:bool)
                n251 = local read "DLL Present"() -> (w255:bool)
                n252 = local write "connect"(w252) -> ()
                n253 = And(x=w255, y=w254) -> (x .and. y?=→"ok for com":bool)
                n254 = local write "start capture"(w252) -> ()
              }
              frame #2 {
                # "put PC-Beamage sync with labview"
                n255 = local read "ok for com"() -> (w256:bool)
                n256 = case shown="True" w256 {
                  frame False {
                  }
                  frame True {
                    w261 = FALSE ("Manual")
                    n257 = local write "Manual"(w261) -> ()
                    n258 = local write "Center :"(enum16{"Centroid", "Peak"}."Centroid" ("Center :")) -> ()
                    n259 = local write "X Axis Measurements"(T3."Centroid" ("X Axis Measurements")) -> ()
                    n260 = local write "subtract background"(w261) -> ()
                    n261 = local write "Orientation :"(enum16{"Auto Orient", "0 Degrees", "45 Degress"}."Auto Orient" ("Orientation :")) -> ()
                    n262 = local write "save current image"(w261) -> ()
                    n263 = local write "Common Measurements"(T4."Measure Effective Diameter" ("Common Measurements")) -> ()
                    n264 = local write "Y Axis Measurements"(T3."Centroid" ("Y Axis Measurements")) -> ()
                    n265 = local write "Display"(T1."3D Display" ("Display")) -> ()
                    n266 = local write "Definition :"(T2."4 Sigma (ISO)" ("Definition :")) -> ()
                    n267 = local write "mm"(200.0 ("mm")) -> ()
                    n268 = local write "Auto"(TRUE ("Auto")) -> ()
                    n269 = property on="save current image" class="Bool (strict)"("DisabledEnum"=T8."Enabled" ("Disabled")) -> ()  [unwired: 2 in, 2 out]
                    n270 = local write "ms"(50.0 ("ms")) -> ()
                    n271 = property on="ms" class="DigNum (strict)"("DisabledEnum"=T8."Disabled and Grayed Out" ("Disabled")) -> ()  [unwired: 2 in, 2 out]
                  }
                }
              }
              frame #3 {
                # "put PC-Beamage sync with labview"
                n272 = local read "ok for com"() -> (w270:bool)
                n273 = case shown="True" w270 {
                  frame False {
                  }
                  frame True {
                    n274 = property on="Common Measurements" class="Enum (strict)"() -> ("RingText.Text"=w273:string)  [unwired: 2 in, 2 out]
                    n275 = Match Pattern(string=w273, regular expression="Measure") -> (after substring=w271:string)  [unwired: 1 in, 3 out]
                    n276 = property on="Common Measurement" class="Str"("Caption.Text"=w271) -> ()  [unwired: 2 in, 2 out]
                  }
                }
              }
              frame #4 {
                # "put PC-Beamage sync with labview"
                n277 = local read "ok for com"() -> (w274:bool)
                n278 = case shown="True" w274 {
                  frame False {
                  }
                  frame True {
                    n279 = property on="X Axis Measurements" class="Enum (strict)"() -> ("RingText.Text"=w277:string)  [unwired: 2 in, 2 out]
                    n280 = Format Into String(format string="X Axis %s", w277) -> (resulting string=w275:string)  [unwired: 2 in, 1 out]
                    n281 = property on="X Axis Measurement" class="Str"("Caption.Text"=w275) -> ()  [unwired: 2 in, 2 out]
                  }
                }
              }
              frame #5 {
                # "put PC-Beamage sync with labview"
                n282 = local read "ok for com"() -> (w278:bool)
                n283 = case shown="True" w278 {
                  frame False {
                  }
                  frame True {
                    n284 = property on="Y Axis Measurements" class="Enum (strict)"() -> ("RingText.Text"=w281:string)  [unwired: 2 in, 2 out]
                    n285 = Format Into String(format string="Y Axis %s", w281) -> (resulting string=w279:string)  [unwired: 2 in, 1 out]
                    n286 = property on="Y Axis Measurement" class="Str"("Caption.Text"=w279) -> ()  [unwired: 2 in, 2 out]
                  }
                }
              }
              frame #6 {
                # "put PC-Beamage sync with labview"
                n287 = local read "ok for com"() -> (w282:bool)
                n288 = case shown="True" w282 {
                  frame False {
                  }
                  frame True {
                    n289 = call "Control 4 Sigma.vi"() -> ("error out"=w288:errorcluster)  [unwired: 9 in, 2 out]
                    n290 = call "Control Centroid.vi"("error in"=w288) -> ("error out"=w289:errorcluster)  [unwired: 8 in, 2 out]
                    n291 = call "Control Auto.vi"("error in"=w289) -> ("error out"=w287:errorcluster)  [unwired: 8 in, 2 out]
                    n292 = call "Display 3D.vi"("error in"=w287) -> ("error out"=w286:errorcluster)  [unwired: 8 in, 2 out]
                    n293 = call "Activate LIN.vi"("error in"=w286) -> ("error out"=w283:errorcluster)  [unwired: 8 in, 2 out]
                    n294 = call "Control Auto Exposure.vi"("error in"=w283) -> ("error out"=w285:errorcluster)  [unwired: 8 in, 2 out]
                    n295 = local read "ms"() -> (w284:dbl)
                    n296 = call "Send Exposure Time.vi"("error in"=w285, "Exposure Time (ms)"=w284) -> ()  [unwired: 7 in, 3 out]
                  }
                }
              }
            }
          }
          event "start capture": Value Change {
            n297 = event-data() -> ("NewVal"=w290:bool)  [unwired: 1 in]
            n298 = local read "ok for com"() -> (w291:bool)
            n299 = case shown="True" w291 {
              tunnel: w290 -> [_ w294]
              frame False {
                n300 = local write "Time out"(-1 ("Time out")) -> ()
                n301 = One Button Dialog(message="Not connected to PC-Beamage Software") -> ()  [unwired: 1 in, 1 out]
              }
              frame True {
                n302 = case shown="True" w294 {
                  frame False {
                    n303 = stacked-sequence {
                      frame #0 {
                        n304 = call "Control Stop Capture.vi"() -> ("error out"=w295:errorcluster)  [unwired: 9 in, 2 out]
                        n305 = local write "Time out"(-1 ("Time out")) -> ()
                        n306 = call <vilib>:"Simple Error Handler.vi"("error in (no error)"=w295) -> ()  [unwired: 4 in, 5 out]
                      }
                      frame #1 {
                        n307 = property on="save current image" class="Bool (strict)"("DisabledEnum"=T8."Enabled" ("Disabled")) -> ()  [unwired: 2 in, 2 out]
                      }
                    }
                  }
                  frame True {
                    n308 = stacked-sequence {
                      frame #0 {
                        # "every 333ms we will go to time out event and get selected data"
                        n309 = call "Control Start Capture.vi"() -> ("error out"=w298:errorcluster)  [unwired: 9 in, 2 out]
                        n310 = local write "Time out"(333 ("Time out")) -> ()
                        n311 = call <vilib>:"Simple Error Handler.vi"("error in (no error)"=w298) -> ()  [unwired: 4 in, 5 out]
                      }
                      frame #1 {
                        n312 = property on="save current image" class="Bool (strict)"("DisabledEnum"=T8."Disabled and Grayed Out" ("Disabled")) -> ()  [unwired: 2 in, 2 out]
                      }
                    }
                  }
                }
              }
            }
          }
          event "save current image": Value Change {
            n313 = event-data() -> ("NewVal"=w301:bool)  [unwired: 1 in]
            n314 = local read "ok for com"() -> (w302:bool)
            n315 = case shown="False" w302 {
              tunnel: w301 -> [_ w305]
              frame False {
                n316 = local write "Time out"(-1 ("Time out")) -> ()
                n317 = One Button Dialog(message="Not connected to PC-Beamage Software") -> ()  [unwired: 1 in, 1 out]
              }
              frame True {
                n318 = case shown="True" w305 {
                  frame False {
                  }
                  frame True {
                    n319 = stacked-sequence {
                      frame #0 {
                        n320 = case shown="\"BMP\"" "Format Image" {
                          tunnel: [w308 w309 w310] -> w306
                          frame "TXT", Default {
                            n321 = call "Control Save Text.vi"() -> ("error out"=w308:errorcluster)  [unwired: 9 in, 2 out]
                          }
                          frame "JPG" {
                            n322 = call "Control JPG Save.vi"() -> ("error out"=w309:errorcluster)  [unwired: 9 in, 2 out]
                          }
                          frame "BMP" {
                            n323 = call "Control BMP Save.vi"() -> ("error out"=w310:errorcluster)  [unwired: 9 in, 2 out]
                          }
                        }
                        n324 = call <vilib>:"Simple Error Handler.vi"("error in (no error)"=w306) -> ()  [unwired: 4 in, 5 out]
                      }
                      frame #1 {
                        n325 = local write "save current image"(FALSE ("save current image")) -> ()
                      }
                    }
                  }
                }
              }
            }
          }
          event "Auto": Value Change {
            n326 = event-data() -> ("NewVal"=w312:bool)  [unwired: 1 in]
            n327 = local read "ok for com"() -> (w313:bool)
            n328 = case shown="True" w313 {
              tunnel: w312 -> [_ w316]
              frame False {
                n329 = local write "Time out"(-1 ("Time out")) -> ()
                n330 = One Button Dialog(message="Not connected to PC-Beamage Software") -> ()  [unwired: 1 in, 1 out]
              }
              frame True {
                n331 = case shown="True" w316 {
                  frame False {
                    # "can't unclick it, must set manual to set this to false"
                    n332 = local write "Manual"(FALSE ("Manual")) -> ()
                    n333 = local write "Auto"(TRUE ("Auto")) -> ()
                    n334 = property on="ms" class="DigNum (strict)"("DisabledEnum"=T8."Disabled and Grayed Out" ("Disabled")) -> ()  [unwired: 2 in, 2 out]
                  }
                  frame True {
                    n335 = stacked-sequence {
                      frame #0 {
                        n336 = call "Control Auto Exposure.vi"() -> ("error out"=w320:errorcluster)  [unwired: 9 in, 2 out]
                        n337 = call <vilib>:"Simple Error Handler.vi"("error in (no error)"=w320) -> ()  [unwired: 4 in, 5 out]
                      }
                      frame #1 {
                        n338 = local write "Manual"(FALSE ("Manual")) -> ()
                        n339 = property on="ms" class="DigNum (strict)"("DisabledEnum"=T8."Disabled and Grayed Out" ("Disabled")) -> ()  [unwired: 2 in, 2 out]
                      }
                    }
                  }
                }
              }
            }
          }
          event "ms": Value Change {
            n340 = event-data() -> ()  [unwired: 1 in, 1 out]
            n341 = local read "ok for com"() -> (w323:bool)
            n342 = case shown="True" w323 {
              frame False {
                n343 = local write "Time out"(-1 ("Time out")) -> ()
                n344 = One Button Dialog(message="Not connected to PC-Beamage Software") -> ()  [unwired: 1 in, 1 out]
              }
              frame True {
                n345 = call "Send Exposure Time.vi"("Exposure Time (ms)"="ms") -> ("error out"=w326:errorcluster)  [unwired: 8 in, 2 out]
                n346 = call <vilib>:"Simple Error Handler.vi"("error in (no error)"=w326) -> ()  [unwired: 4 in, 5 out]
              }
            }
          }
          event "mm": Value Change {
            n347 = event-data() -> ()  [unwired: 1 in, 1 out]
            n348 = local read "ok for com"() -> (w328:bool)
            n349 = case shown="False" w328 {
              frame False {
                n350 = local write "Time out"(-1 ("Time out")) -> ()
                n351 = One Button Dialog(message="Not connected to PC-Beamage Software") -> ()  [unwired: 1 in, 1 out]
              }
              frame True {
                n352 = call "Send Focal Length Divergence.vi"("Focal Length"="mm") -> ("error out"=w332:errorcluster)  [unwired: 8 in, 2 out]
                n353 = call <vilib>:"Simple Error Handler.vi"("error in (no error)"=w332) -> ()  [unwired: 4 in, 5 out]
              }
            }
          }
          event "Gray Scale": Value Change {
            n354 = event-data() -> ()  [unwired: 1 in, 6 out]
            n355 = local read "ok for com"() -> (w333:bool)
            n356 = case shown="False" w333 {
              frame False {
                n357 = stacked-sequence {
                  frame #0 {
                    n358 = One Button Dialog(message="Not connected to PC-Beamage Software") -> ()  [unwired: 1 in, 1 out]
                  }
                  frame #1 {
                    n359 = local write "Gray Scale"(FALSE ("Gray Scale")) -> ()
                    n360 = local write "Time out"(-1 ("Time out")) -> ()
                  }
                }
              }
              frame True {
                n361 = call "Activate Gray Scale.vi"() -> ("error out"=w337:errorcluster)  [unwired: 9 in, 2 out]
                n362 = call <vilib>:"Simple Error Handler.vi"("error in (no error)"=w337) -> ()  [unwired: 4 in, 5 out]
              }
            }
          }
          event "subtract background": Value Change {
            n363 = event-data() -> ("NewVal"=w338:bool)  [unwired: 1 in]
            n364 = local read "ok for com"() -> (w339:bool)
            n365 = case shown="True" w339 {
              tunnel: w338 -> [_ w342]
              frame False {
                n366 = local write "Time out"(-1 ("Time out")) -> ()
                n367 = One Button Dialog(message="Not connected to PC-Beamage Software") -> ()  [unwired: 1 in, 1 out]
              }
              frame True {
                n368 = case shown="True" w342 {
                  frame False {
                    n369 = call "Deactivate Subtract Background.vi"() -> ("error out"=w343:errorcluster)  [unwired: 9 in, 2 out]
                    n370 = call <vilib>:"Simple Error Handler.vi"("error in (no error)"=w343) -> ()  [unwired: 4 in, 5 out]
                  }
                  frame True {
                    n371 = local read "start capture"() -> (w344:bool)
                    n372 = case shown="True" w344 {
                      frame False {
                        n373 = local write "subtract background"(FALSE ("subtract background")) -> ()
                        n374 = One Button Dialog(message="Please press Start Capture to enable the subtract background function.") -> ()  [unwired: 1 in, 1 out]
                      }
                      frame True {
                        n375 = stacked-sequence {
                          seq-local: [w347 _ _] -> [_ w349 _]
                          frame #0 {
                            n376 = Two Button Dialog(message="Please Block your laser ") -> (T button?=w347:bool)  [unwired: 2 in]
                          }
                          frame #1 {
                            n377 = case shown="True" w349 {
                              frame False {
                              }
                              frame True {
                                n378 = call "Activate Subtract Background.vi"() -> ("error out"=w350:errorcluster)  [unwired: 9 in, 2 out]
                                n379 = call <vilib>:"Simple Error Handler.vi"("error in (no error)"=w350) -> ()  [unwired: 4 in, 5 out]
                              }
                            }
                          }
                          frame #2 {
                          }
                        }
                      }
                    }
                  }
                }
              }
            }
          }
          event "Manual": Value Change {
            n380 = event-data() -> ("NewVal"=w351:bool)  [unwired: 1 in]
            n381 = local read "ok for com"() -> (w352:bool)
            n382 = case shown="True" w352 {
              tunnel: w351 -> [_ w355]
              frame False {
                n383 = local write "Time out"(-1 ("Time out")) -> ()
                n384 = One Button Dialog(message="Not connected to PC-Beamage Software") -> ()  [unwired: 1 in, 1 out]
              }
              frame True {
                n385 = case shown="True" w355 {
                  frame False {
                    # "can't unclick it, must set auto to set this to false"
                    n386 = local write "Manual"(TRUE ("Manual")) -> ()
                    n387 = local write "Auto"(FALSE ("Auto")) -> ()
                    n388 = property on="ms" class="DigNum (strict)"("DisabledEnum"=T8."Enabled" ("Disabled")) -> ()  [unwired: 2 in, 2 out]
                  }
                  frame True {
                    n389 = stacked-sequence {
                      frame #0 {
                        n390 = call "Control Manual Exposure.vi"() -> ("error out"=w360:errorcluster)  [unwired: 9 in, 2 out]
                        n391 = local read "ms"() -> (w361:dbl)
                        n392 = call "Send Exposure Time.vi"("error in"=w360, "Exposure Time (ms)"=w361) -> ("error out"=w359:errorcluster)  [unwired: 7 in, 2 out]
                        n393 = call <vilib>:"Simple Error Handler.vi"("error in (no error)"=w359) -> ()  [unwired: 4 in, 5 out]
                      }
                      frame #1 {
                        n394 = local write "Auto"(FALSE ("Manual")) -> ()
                        n395 = property on="ms" class="DigNum (strict)"("DisabledEnum"=T8."Enabled" ("Disabled")) -> ()  [unwired: 2 in, 2 out]
                      }
                    }
                  }
                }
              }
            }
          }
          event "Definition :": Value Change {
            n396 = event-data() -> ("NewVal"=w364:T2)  [unwired: 1 in]
            n397 = local read "ok for com"() -> (w365:bool)
            n398 = case shown="True" w365 {
              tunnel: w364 -> [_ w367]
              frame False {
                n399 = One Button Dialog(message="Not connected to PC-Beamage Software") -> ()  [unwired: 1 in, 1 out]
              }
              frame True {
                n400 = case shown="\"FWHM along Crosshairs (50%)\"" w367 {
                  frame "4 Sigma (ISO)", Default {
                    n401 = call "Control 4 Sigma.vi"() -> ("error out"=w368:errorcluster)  [unwired: 9 in, 2 out]
                    n402 = call <vilib>:"Simple Error Handler.vi"("error in (no error)"=w368) -> ()  [unwired: 4 in, 5 out]
                  }
                  frame "FWHM along Crosshairs (50%)" {
                    n403 = call "Control FWHM.vi"() -> ("error out"=w369:errorcluster)  [unwired: 9 in, 2 out]
                    n404 = call <vilib>:"Simple Error Handler.vi"("error in (no error)"=w369) -> ()  [unwired: 4 in, 5 out]
                  }
                  frame "1 / e^2 along Crosshairs (13.5%)" {
                    n405 = call "Control 1OVRe^2.vi"() -> ("error out"=w370:errorcluster)  [unwired: 9 in, 2 out]
                    n406 = call <vilib>:"Simple Error Handler.vi"("error in (no error)"=w370) -> ()  [unwired: 4 in, 5 out]
                  }
                  frame "86 % effective Diameter" {
                    n407 = call "Control 86.vi"() -> ("error out"=w371:errorcluster)  [unwired: 9 in, 2 out]
                    n408 = call <vilib>:"Simple Error Handler.vi"("error in (no error)"=w371) -> ()  [unwired: 4 in, 5 out]
                  }
                }
              }
            }
          }
          event "Display": Value Change {
            n409 = event-data() -> ("NewVal"=w373:T1)  [unwired: 1 in]
            n410 = local read "ok for com"() -> (w374:bool)
            n411 = case shown="False" w374 {
              tunnel: w373 -> [_ w378]
              tunnel: [FALSE ("Visible") w377] -> w372
              frame False {
                n412 = One Button Dialog(message="Not connected to PC-Beamage Software") -> ()  [unwired: 1 in, 1 out]
              }
              frame True {
                n413 = case shown="\"Beam Track Display\"" w378 {
                  tunnel: [FALSE ("Visible") FALSE ("Visible") TRUE ("Visible") FALSE ("Visible")] -> w377
                  frame "2D Display", Default {
                    w379 = FALSE ("Visible")
                    n414 = call "Display 2D.vi"() -> ("error out"=w381:errorcluster)  [unwired: 9 in, 2 out]
                    n415 = call <vilib>:"Simple Error Handler.vi"("error in (no error)"=w381) -> ()  [unwired: 4 in, 5 out]
                    n416 = property on="FWHM On" class="Bool (strict)"("Visible"=w379) -> ()  [unwired: 2 in, 2 out]
                    n417 = property on="Log on" class="Bool (strict)"("Visible"=w379) -> ()  [unwired: 2 in, 2 out]
                    n418 = property on="Gauss on" class="Bool (strict)"("Visible"=w379) -> ()  [unwired: 2 in, 2 out]
                    n419 = property on="1ovre on" class="Bool (strict)"("Visible"=w379) -> ()  [unwired: 2 in, 2 out]
                  }
                  frame "3D Display" {
                    w382 = FALSE ("Visible")
                    n420 = call "Display 3D.vi"() -> ("error out"=w384:errorcluster)  [unwired: 9 in, 2 out]
                    n421 = call <vilib>:"Simple Error Handler.vi"("error in (no error)"=w384) -> ()  [unwired: 4 in, 5 out]
                    n422 = property on="FWHM On" class="Bool (strict)"("Visible"=w382) -> ()  [unwired: 2 in, 2 out]
                    n423 = property on="Log on" class="Bool (strict)"("Visible"=w382) -> ()  [unwired: 2 in, 2 out]
                    n424 = property on="Gauss on" class="Bool (strict)"("Visible"=w382) -> ()  [unwired: 2 in, 2 out]
                    n425 = property on="1ovre on" class="Bool (strict)"("Visible"=w382) -> ()  [unwired: 2 in, 2 out]
                  }
                  frame "XY Display" {
                    w385 = FALSE ("Visible")
                    n426 = call "Display XY.vi"() -> ("error out"=w387:errorcluster)  [unwired: 9 in, 2 out]
                    n427 = call <vilib>:"Simple Error Handler.vi"("error in (no error)"=w387) -> ()  [unwired: 4 in, 5 out]
                    n428 = property on="FWHM On" class="Bool (strict)"("Visible"=w385) -> ()  [unwired: 2 in, 2 out]
                    n429 = property on="Log on" class="Bool (strict)"("Visible"=w385) -> ()  [unwired: 2 in, 2 out]
                    n430 = property on="Gauss on" class="Bool (strict)"("Visible"=w385) -> ()  [unwired: 2 in, 2 out]
                    n431 = property on="1ovre on" class="Bool (strict)"("Visible"=w385) -> ()  [unwired: 2 in, 2 out]
                  }
                  frame "Beam Track Display" {
                    w388 = FALSE ("Visible")
                    n432 = call "Display TRACK.vi"() -> ("error out"=w390:errorcluster)  [unwired: 9 in, 2 out]
                    n433 = call <vilib>:"Simple Error Handler.vi"("error in (no error)"=w390) -> ()  [unwired: 4 in, 5 out]
                    n434 = property on="FWHM On" class="Bool (strict)"("Visible"=w388) -> ()  [unwired: 2 in, 2 out]
                    n435 = property on="Log on" class="Bool (strict)"("Visible"=w388) -> ()  [unwired: 2 in, 2 out]
                    n436 = property on="Gauss on" class="Bool (strict)"("Visible"=w388) -> ()  [unwired: 2 in, 2 out]
                    n437 = property on="1ovre on" class="Bool (strict)"("Visible"=w388) -> ()  [unwired: 2 in, 2 out]
                  }
                }
              }
            }
            n438 = property on="Display" class="Enum (strict)"("Caption.Visible"=w372) -> ()  [unwired: 2 in, 2 out]
            n439 = property on="Log" class="Bool (strict)"("Visible"=w372) -> ()  [unwired: 2 in, 2 out]
            n440 = property on="Gauss" class="Bool (strict)"("Visible"=w372) -> ()  [unwired: 2 in, 2 out]
            n441 = property on="FWHM" class="Bool (strict)"("Visible"=w372) -> ()  [unwired: 2 in, 2 out]
            n442 = property on="1ovre" class="Bool (strict)"("Visible"=w372) -> ()  [unwired: 2 in, 2 out]
          }
          event "Center :": Value Change {
            n443 = event-data() -> ("NewVal"=w391:enum16{"Centroid", "Peak"})  [unwired: 1 in]
            n444 = local read "ok for com"() -> (w392:bool)
            n445 = case shown="False" w392 {
              tunnel: w391 -> [_ w394]
              frame False {
                n446 = One Button Dialog(message="Not connected to PC-Beamage Software") -> ()  [unwired: 1 in, 1 out]
              }
              frame True {
                n447 = case shown="\"Centroid\", Default" w394 {
                  frame "Centroid", Default {
                    n448 = call "Control Centroid.vi"() -> ("error out"=w395:errorcluster)  [unwired: 9 in, 2 out]
                    n449 = call <vilib>:"Simple Error Handler.vi"("error in (no error)"=w395) -> ()  [unwired: 4 in, 5 out]
                  }
                  frame "Peak" {
                    n450 = call "Control Peak.vi"() -> ("error out"=w396:errorcluster)  [unwired: 9 in, 2 out]
                    n451 = call <vilib>:"Simple Error Handler.vi"("error in (no error)"=w396) -> ()  [unwired: 4 in, 5 out]
                  }
                }
              }
            }
          }
          event "Gauss": Value Change {
            n452 = event-data() -> ("NewVal"=w397:bool)  [unwired: 1 in]
            n453 = local read "ok for com"() -> (w398:bool)
            n454 = case shown="False" w398 {
              tunnel: w397 -> [_ w401]
              frame False {
                w399 = FALSE ("verifiy dll")
                n455 = local write "Gauss"(w399) -> ()
                n456 = local write "Gauss on"(w399) -> ()
                n457 = One Button Dialog(message="Not connected to PC-Beamage Software") -> ()  [unwired: 1 in, 1 out]
              }
              frame True {
                n458 = case shown="True" w401 {
                  frame False {
                  }
                  frame True {
                    n459 = local write "Gauss on"(FALSE ("Gauss on")) -> ()
                    n460 = property on="Gauss on" class="Bool (strict)"("Visible"=TRUE) -> ()  [unwired: 2 in, 2 out]
                    n461 = property on="Gauss" class="Bool (strict)"("Visible"=FALSE) -> ()  [unwired: 2 in, 2 out]
                    n462 = call "Activate Gaussian.vi"() -> ()  [unwired: 9 in, 3 out]
                  }
                }
              }
            }
          }
          event "Log": Value Change {
            n463 = event-data() -> ("NewVal"=w405:bool)  [unwired: 1 in]
            n464 = local read "ok for com"() -> (w406:bool)
            n465 = case shown="False" w406 {
              tunnel: w405 -> [_ w409]
              frame False {
                w407 = FALSE ("verifiy dll")
                n466 = local write "Log on"(w407) -> ()
                n467 = local write "Log"(w407) -> ()
                n468 = One Button Dialog(message="Not connected to PC-Beamage Software") -> ()  [unwired: 1 in, 1 out]
              }
              frame True {
                n469 = case shown="True" w409 {
                  frame False {
                  }
                  frame True {
                    n470 = local write "Log on"(FALSE ("Gauss on")) -> ()
                    n471 = property on="Log on" class="Bool (strict)"("Visible"=TRUE) -> ()  [unwired: 2 in, 2 out]
                    n472 = property on="Log" class="Bool (strict)"("Visible"=FALSE) -> ()  [unwired: 2 in, 2 out]
                    n473 = call "Activate LOG.vi"() -> ()  [unwired: 9 in, 3 out]
                  }
                }
              }
            }
          }
          event "FWHM": Value Change {
            n474 = event-data() -> ("NewVal"=w413:bool)  [unwired: 1 in]
            n475 = local read "ok for com"() -> (w414:bool)
            n476 = case shown="False" w414 {
              tunnel: w413 -> [_ w417]
              frame False {
                w415 = FALSE ("verifiy dll")
                n477 = local write "FWHM On"(w415) -> ()
                n478 = local write "FWHM"(w415) -> ()
                n479 = One Button Dialog(message="Not connected to PC-Beamage Software") -> ()  [unwired: 1 in, 1 out]
              }
              frame True {
                n480 = case shown="True" w417 {
                  frame False {
                  }
                  frame True {
                    n481 = local write "FWHM On"(FALSE ("Gauss on")) -> ()
                    n482 = property on="FWHM On" class="Bool (strict)"("Visible"=TRUE) -> ()  [unwired: 2 in, 2 out]
                    n483 = property on="FWHM" class="Bool (strict)"("Visible"=FALSE) -> ()  [unwired: 2 in, 2 out]
                    n484 = call "Activate FWHM.vi"() -> ()  [unwired: 9 in, 3 out]
                  }
                }
              }
            }
          }
          event "1ovre": Value Change {
            n485 = event-data() -> ("NewVal"=w421:bool)  [unwired: 1 in]
            n486 = local read "ok for com"() -> (w422:bool)
            n487 = case shown="False" w422 {
              tunnel: w421 -> [_ w425]
              frame False {
                w423 = FALSE ("verifiy dll")
                n488 = local write "1ovre on"(w423) -> ()
                n489 = local write "1ovre"(w423) -> ()
                n490 = One Button Dialog(message="Not connected to PC-Beamage Software") -> ()  [unwired: 1 in, 1 out]
              }
              frame True {
                n491 = case shown="True" w425 {
                  frame False {
                  }
                  frame True {
                    n492 = local write "1ovre on"(FALSE ("Gauss on")) -> ()
                    n493 = property on="1ovre on" class="Bool (strict)"("Visible"=TRUE) -> ()  [unwired: 2 in, 2 out]
                    n494 = property on="1ovre" class="Bool (strict)"("Visible"=FALSE) -> ()  [unwired: 2 in, 2 out]
                    n495 = call "Activate 1OVRE.vi"() -> ()  [unwired: 9 in, 3 out]
                  }
                }
              }
            }
          }
          event "Gauss on": Value Change {
            n496 = event-data() -> ("NewVal"=w429:bool)  [unwired: 1 in]
            n497 = local read "ok for com"() -> (w430:bool)
            n498 = case shown="True" w430 {
              tunnel: w429 -> [_ w433]
              frame False {
                w431 = FALSE ("verifiy dll")
                n499 = local write "Gauss"(w431) -> ()
                n500 = local write "Gauss on"(w431) -> ()
                n501 = One Button Dialog(message="Not connected to PC-Beamage Software") -> ()  [unwired: 1 in, 1 out]
              }
              frame True {
                n502 = case shown="False" w433 {
                  frame False {
                  }
                  frame True {
                    n503 = local write "Gauss"(FALSE ("Gauss")) -> ()
                    n504 = property on="Gauss" class="Bool (strict)"("Visible"=TRUE) -> ()  [unwired: 2 in, 2 out]
                    n505 = property on="Gauss on" class="Bool (strict)"("Visible"=FALSE) -> ()  [unwired: 2 in, 2 out]
                  }
                }
              }
            }
          }
          event "Log on": Value Change {
            n506 = event-data() -> ("NewVal"=w437:bool)  [unwired: 1 in]
            n507 = local read "ok for com"() -> (w438:bool)
            n508 = case shown="False" w438 {
              tunnel: w437 -> [_ w441]
              frame False {
                w439 = FALSE ("verifiy dll")
                n509 = local write "Log"(w439) -> ()
                n510 = local write "Log on"(w439) -> ()
                n511 = One Button Dialog(message="Not connected to PC-Beamage Software") -> ()  [unwired: 1 in, 1 out]
              }
              frame True {
                n512 = case shown="True" w441 {
                  frame False {
                  }
                  frame True {
                    n513 = local write "Log"(FALSE ("Gauss")) -> ()
                    n514 = property on="Log" class="Bool (strict)"("Visible"=TRUE) -> ()  [unwired: 2 in, 2 out]
                    n515 = property on="Log on" class="Bool (strict)"("Visible"=FALSE) -> ()  [unwired: 2 in, 2 out]
                    n516 = call "Activate LIN.vi"() -> ()  [unwired: 9 in, 3 out]
                  }
                }
              }
            }
          }
          event "FWHM On": Value Change {
            n517 = event-data() -> ("NewVal"=w445:bool)  [unwired: 1 in]
            n518 = local read "ok for com"() -> (w446:bool)
            n519 = case shown="False" w446 {
              tunnel: w445 -> [_ w449]
              frame False {
                w447 = FALSE ("verifiy dll")
                n520 = local write "FWHM On"(w447) -> ()
                n521 = local write "FWHM"(w447) -> ()
                n522 = One Button Dialog(message="Not connected to PC-Beamage Software") -> ()  [unwired: 1 in, 1 out]
              }
              frame True {
                n523 = case shown="True" w449 {
                  frame False {
                  }
                  frame True {
                    n524 = local write "FWHM"(FALSE ("Gauss")) -> ()
                    n525 = property on="FWHM" class="Bool (strict)"("Visible"=TRUE) -> ()  [unwired: 2 in, 2 out]
                    n526 = property on="FWHM On" class="Bool (strict)"("Visible"=FALSE) -> ()  [unwired: 2 in, 2 out]
                  }
                }
              }
            }
          }
          event "1ovre on": Value Change {
            n527 = event-data() -> ("NewVal"=w453:bool)  [unwired: 1 in]
            n528 = local read "ok for com"() -> (w454:bool)
            n529 = case shown="False" w454 {
              tunnel: w453 -> [_ w457]
              frame False {
                w455 = FALSE ("verifiy dll")
                n530 = local write "1ovre on"(w455) -> ()
                n531 = local write "1ovre"(w455) -> ()
                n532 = One Button Dialog(message="Not connected to PC-Beamage Software") -> ()  [unwired: 1 in, 1 out]
              }
              frame True {
                n533 = case shown="True" w457 {
                  frame False {
                  }
                  frame True {
                    n534 = local write "1ovre"(FALSE ("Gauss")) -> ()
                    n535 = property on="1ovre" class="Bool (strict)"("Visible"=TRUE) -> ()  [unwired: 2 in, 2 out]
                    n536 = property on="1ovre on" class="Bool (strict)"("Visible"=FALSE) -> ()  [unwired: 2 in, 2 out]
                  }
                }
              }
            }
          }
          event "Common Measurements": Value Change {
            n537 = event-data() -> ("NewVal"=w461:T4)  [unwired: 1 in]
            n538 = local read "ok for com"() -> (w462:bool)
            n539 = case shown="False" w462 {
              tunnel: w461 -> [_ _]
              frame False {
                n540 = One Button Dialog(message="Not connected to PC-Beamage Software") -> ()  [unwired: 1 in, 1 out]
              }
              frame True {
                n541 = property on="Common Measurements" class="Enum (strict)"() -> ("RingText.Text"=w466:string)  [unwired: 2 in, 2 out]
                n542 = Match Pattern(string=w466, regular expression="Measure") -> (after substring=w464:string)  [unwired: 1 in, 3 out]
                n543 = property on="Common Measurement" class="Str"("Caption.Text"=w464) -> ()  [unwired: 2 in, 2 out]
              }
            }
          }
          event "X Axis Measurements": Value Change {
            n544 = event-data() -> ("NewVal"=w467:T3)  [unwired: 1 in]
            n545 = local read "ok for com"() -> (w468:bool)
            n546 = case shown="False" w468 {
              tunnel: w467 -> [_ w471]
              frame False {
                n547 = One Button Dialog(message="Not connected to PC-Beamage Software") -> ()  [unwired: 1 in, 1 out]
              }
              frame True {
                n548 = property on="X Axis Measurements" class="Enum (strict)"() -> ("RingText.Text"=w474:string)  [unwired: 2 in, 2 out]
                n549 = case shown="\"1/e^2\", Default" w471 {
                  tunnel: [u32 35 ("Text.Font:Size") u32 20 ("Text.Font:Size")] -> w470
                  frame "1/e^2", Default {
                  }
                  frame "Gaussian Equation" {
                  }
                }
                n550 = Format Into String(format string="X Axis %s", w474) -> (resulting string=w472:string)  [unwired: 2 in, 1 out]
                n551 = property on="X Axis Measurement" class="Str"("Caption.Text"=w472) -> ()  [unwired: 2 in, 2 out]
                n552 = property on="X Axis Measurement" class="Str"("Text.FontSize"=w470) -> ()  [unwired: 2 in, 2 out]
              }
            }
          }
          event "Y Axis Measurements": Value Change {
            n553 = event-data() -> ("NewVal"=w477:T3)  [unwired: 1 in]
            n554 = local read "ok for com"() -> (w478:bool)
            n555 = case shown="False" w478 {
              tunnel: w477 -> [_ w481]
              frame False {
                n556 = One Button Dialog(message="Not connected to PC-Beamage Software") -> ()  [unwired: 1 in, 1 out]
              }
              frame True {
                n557 = property on="Y Axis Measurements" class="Enum (strict)"() -> ("RingText.Text"=w484:string)  [unwired: 2 in, 2 out]
                n558 = case shown="\"Gaussian Equation\"" w481 {
                  tunnel: [u32 35 ("Text.Font:Size") u32 20 ("Text.Font:Size")] -> w480
                  frame "1/e^2", Default {
                  }
                  frame "Gaussian Equation" {
                  }
                }
                n559 = Format Into String(format string="Y Axis %s", w484) -> (resulting string=w482:string)  [unwired: 2 in, 1 out]
                n560 = property on="Y Axis Measurement" class="Str"("Caption.Text"=w482) -> ()  [unwired: 2 in, 2 out]
                n561 = property on="Y Axis Measurement" class="Str"("Text.FontSize"=w480) -> ()  [unwired: 2 in, 2 out]
              }
            }
          }
          event "Orientation :": Value Change {
            n562 = event-data() -> ("NewVal"=w487:enum16{"Auto Orient", "0 Degrees", "45 Degress"})  [unwired: 1 in]
            n563 = local read "ok for com"() -> (w488:bool)
            n564 = case shown="False" w488 {
              tunnel: w487 -> [_ w490]
              frame False {
                n565 = One Button Dialog(message="Not connected to PC-Beamage Software") -> ()  [unwired: 1 in, 1 out]
              }
              frame True {
                n566 = case shown="\"Auto Orient\", Default" w490 {
                  frame "Auto Orient", Default {
                    n567 = call "Control Auto.vi"() -> ("error out"=w491:errorcluster)  [unwired: 9 in, 2 out]
                    n568 = call <vilib>:"Simple Error Handler.vi"("error in (no error)"=w491) -> ()  [unwired: 4 in, 5 out]
                  }
                  frame "0 Degrees" {
                    n569 = call "Control Zero.vi"() -> ("error out"=w492:errorcluster)  [unwired: 9 in, 2 out]
                    n570 = call <vilib>:"Simple Error Handler.vi"("error in (no error)"=w492) -> ()  [unwired: 4 in, 5 out]
                  }
                  frame "45 Degress" {
                    n571 = call "Control 45.vi"() -> ("error out"=w493:errorcluster)  [unwired: 9 in, 2 out]
                    n572 = call <vilib>:"Simple Error Handler.vi"("error in (no error)"=w493) -> ()  [unwired: 4 in, 5 out]
                  }
                }
              }
            }
          }
          event "Divergence Button": Value Change {
            n573 = event-data() -> ()  [unwired: 1 in, 1 out]
            n574 = case shown="False" "Divergence Button" {
              frame False {
                n575 = call "Activate Divergence.vi"() -> ("error out"=w496:errorcluster)  [unwired: 9 in, 2 out]
                n576 = call <vilib>:"Simple Error Handler.vi"("error in (no error)"=w496) -> ()  [unwired: 4 in, 5 out]
                n577 = property on="mm" class="DigNum (strict)"("DisabledEnum"=T8."Disabled and Grayed Out" ("Disabled")) -> ()  [unwired: 2 in, 2 out]
              }
              frame True {
                n578 = call "Activate Divergence.vi"() -> ("error out"=w498:errorcluster)  [unwired: 9 in, 2 out]
                n579 = call <vilib>:"Simple Error Handler.vi"("error in (no error)"=w498) -> ()  [unwired: 4 in, 5 out]
                n580 = property on="mm" class="DigNum (strict)"("DisabledEnum"=T8."Enabled" ("Disabled")) -> ()  [unwired: 2 in, 2 out]
              }
            }
          }
          event "disconnect": Value Change {
            n581 = event-data() -> ()  [unwired: 1 in, 1 out]
            n582 = stacked-sequence {
              frame #0 {
                n583 = local read "Connected"() -> (w499:bool)
                n584 = case shown="False" w499 {
                  frame False {
                    n585 = One Button Dialog(message="Not Connected") -> ()  [unwired: 1 in, 1 out]
                  }
                  frame True {
                    n586 = call "Control Stop Capture.vi"() -> ("error out"=w501:errorcluster)  [unwired: 9 in, 2 out]
                    n587 = call "Disconnect PC Beamage 64 Bit DLL.vi"("error in"=w501) -> ("error out"=w504:errorcluster, "Disconnected"=w503:bool)  [unwired: 9 in]
                    n588 = Not(x=w503) -> (.not. x?=w502:bool)
                    n589 = local write "Connected"(w502) -> ()
                    n590 = call <vilib>:"Simple Error Handler.vi"("error in (no error)"=w504) -> ()  [unwired: 4 in, 5 out]
                  }
                }
              }
              frame #1 {
                w505 = FALSE ("verifiy dll")
                n591 = local write "disconnect"(w505) -> ()
                n592 = local write "Time out"(-1 ("Time out")) -> ()
                n593 = local write "start capture"(w505) -> ()
              }
            }
          }
          event "exit": Value Change {
            n594 = event-data() -> ()  [unwired: 1 in, 1 out]
            n595 = flat-sequence {
              frame #0 {
                n596 = local read "Connected"() -> (w507:bool)
                n597 = case shown="True" w507 {
                  frame False {
                  }
                  frame True {
                    n598 = call "Control Stop Capture.vi"() -> ("error out"=w509:errorcluster)  [unwired: 9 in, 2 out]
                    n599 = call "Disconnect PC Beamage 64 Bit DLL.vi"("error in"=w509) -> ("error out"=w508:errorcluster, "Disconnected"=w511:bool)  [unwired: 9 in]
                    n600 = Not(x=w511) -> (.not. x?=w510:bool)
                    n601 = local write "Connected"(w510) -> ()
                    n602 = call <vilib>:"Simple Error Handler.vi"("error in (no error)"=w508) -> ()  [unwired: 4 in, 5 out]
                  }
                }
              }
              frame #1 {
                w514 = FALSE ("verifiy dll")
                n603 = local write "start capture"(FALSE ("stop capture")) -> ()
                n604 = local write "DLL Present"(w514) -> ()
                n605 = local write "exit"(w514) -> ()
                n606 = property on="start capture" class="Bool (strict)"("Visible"=TRUE) -> ()  [unwired: 2 in, 2 out]
              }
              frame #2 {
                n607 = call "Stay or Go.vi"() -> ()  [unwired: 12 in]
              }
            }
          }
        }
      }
    }
  }
  n608 = while {
    stop <- "stop" stop-if-true
    n609 = call <vilib>:"Read BMP File.vi"("path to BMP file"=path "C:/Users/Ford/Documents/Gentec-EO/beamage.bmp") -> ("image data"=w518:T7)  [unwired: 8 in, 2 out]
    n610 = call <vilib>:"Draw Flattened Pixmap.vi"("image data"=w518) -> ("new picture"=→"new picture":picture)  [unwired: 8 in]
  }
